vi "eyecat MAX v02_test.vi"() -> ()   [LabVIEW 2014]
doc: "This VI is an upgrade from the WIN 1_v4 that implements the ageing subrutine"
uses:
  Buttons/String output.ctl
  <vilib>/Utility/miscctls.llb/LVRowAndColumnTypeDef.ctl
  Buttons/Numeric control.ctl
  Buttons/String input.ctl
  Buttons/Numeric indicator.ctl
  Controls Win/Control 3.ctl
  <vilib>/Platform/TimedLoop/XDataNode/nitl_modes.ctl
  <vilib>/Platform/TimedLoop/XDataNode/timing_clust.ctl
  <vilib>/Platform/TimedLoop/XDataNode/wakeup.ctl
  <vilib>/Utility/file.llb/Read From Spreadsheet File (DBL).vi
  <vilib>/Utility/file.llb/Write To Spreadsheet File (string).vi
  <vilib>/Utility/file.llb/Read From Spreadsheet File (string).vi
  <vilib>/regexp/Match Regular Expression.xnode
  <vilib>/Platform/TimedLoop/XDataNode/XDataNode.xnode
  <vilib>/Platform/TimedLoop/XDataNode/XDNodeRunTimeDep.lvlib
panel:
  out "output cluster":T2
  out "Lambda":dbl[](array[numeric])
  out "MKS HC":dbl
  in  "HC Index":i32
  in  "MFC Number":i32
  out "Open/Closed Loop array":dbl[](array[numeric])
  out "Air Cyc 2 array":dbl[](array[numeric])
  in  "Cycle size":i32
  out "MFC Setpoint/Delivery":dynamicdata(graph)
  out "ExtAnDn":bool
  out "ExtAnUp":bool
  out "HC Cyc 2 Array":dbl[](array[numeric])
  out "SO Valve 2 array":dbl[](array[numeric])
  out "SO Valve 1 array":dbl[](array[numeric])
  out "Air Bal array":dbl[](array[numeric])
  out "HC Bal array":dbl[](array[numeric])
  out "Air Cyc 1 array":dbl[](array[numeric])
  out "HC Cyc 1 array":dbl[](array[numeric])
  out "File name":string
  out "Log?":bool
  out "Advanced Logging":bool
  out "Connected":bool
  out "MKS 1":i16
  out "MKS 2":i16
  out "Furnace temp 2":dbl
  out "Full system?":bool
  out "Log interval (seconds)":T1
  in  "Flow rate Age":dbl
  in  "Inlet temp Age":dbl
  out "Stopped?":bool
  in  "Stop Cmd":T1
  out "Connected?":bool
  out "Error":dbl
  out "Iteration Duration":i64
  out "Finished Late? [i-1]":bool
  in  "stop TCP":bool
  in  "SO2 ppm":dbl
  out "Furnace temp 1":dbl
  out "stop 2":bool
  in  "Enum 1":i16=1
  in  "Acknowledge":bool
  out "Test number":u16
  out "Flag1":bool=TRUE
  out "EditPos Subc":T3
  out "Flag 2":bool=TRUE
  in  "Tab Control":T4(tab)
  out "Doors Unlocked":bool
  in  "Temperature Limit (°C)":T1=800.0 min=0.0 max=1200.0 step=1.0
  in  "Log Test Button":bool
  in  "File Name":T5="Test"
  in  "File Path":path=path "C:/DATA LOG"
  out "Fail":bool
  out "Pass":bool
  in  "Select Test Type":T6(radio)
  out "Standby":bool
  out "Doors Open":bool
  out "Extractor Fan On":bool
  out "Test In Progress":bool
  out "Cool Down":bool
  out "System Alarm":bool
  in  "Execute Leak Test Button":bool
  in  "Stop Test Button":bool
  in  "Start Test Button":bool
  in  "Advanced settings":bool
  in  "Inlet Temperature (°C)":T1=400.0 min=350.0 max=1000.0 step=1.0
  in  "Inlet LAMBDA Rich":T1=0.9 min=0.85 max=0.96 step=0.001
  in  "Inlet LAMBDA Lean":T1=1.2 min=1.02 max=3.0 step=0.001
  in  "Test Stop temperature (°C)":T1=300.0 min=100.0 max=1000.0 step=1.0
  in  "Test Start Temperature (°C)":T1=125.0 min=0.0 max=500.0 step=1.0
  in  "Furnace Ramp Rate (°C/min)":T1=15.0 min=1.0 max=50.0 step=0.1
  in  "NO:CO Ratio":T1=1.1 min=1.0 max=5.0 step=0.1
  in  "Inlet O2 (%)":T1=0.5 min=0.0 max=14.0 step=0.01
  in  "Inlet LAMBDA":T1=1.0 min=0.6 max=3.0 step=0.001
  out "Space Velocity (h-1)":T7
  out "Vol Flow @ STP (l/min)":T7
  in  "Test Flow Rate(g/s)":T1 min=0.0 max=100.0 step=0.01
  out "Sample Volume (litres)":T7
  in  "Number of Samples":T1=1.0 min=1.0 max=6.0 step=1.0
  in  "Sample Diameter (mm)":T1
  out "CO Theory (%)":T7 format="%#_3g"
  out "CO Theory (%)":T7 format="%#_3g"
  out "HC Theory (%)":T7
  in  "Sample Length (mm)":T1 min=0.0 step=0.5
  in  "NO ppm SW":dbl=500.0 caption="NO (ppm)" min=0.0 max=500.0 step=1.0
  in  "NO ppm Loff":T1 caption="NO ppm"
  in  "Delete sCycle":bool
  in  "Load sCycle":bool
  in  "Save sCycle":bool
  in  "Clear subcycle":bool
  in  "Clear Cycle Pattern":bool
  in  "Save Cycle":bool
  in  "Load Cycle":bool
  in  "Delete Cycle":bool
  out "Test Compiled":bool
  in  "Compile Test Button":bool
  in  "Sub-Cycle List":i32(listbox)=1
  in  "Cycle List":i32(listbox)=2
  out "Total Test Duration (hrs)":T8
  in  "Ageing Gas":enum32{"Radio Selection 1", "Radio Selection 2"}(radio)
  in  "Sub-Cycle Pattern":string[][](table) caption="Subcycle pattern"
  in  "Total Number of Cycles":T1=1.0 min=1.0 max=10000.0 step=1.0
  in  "Cycle Pattern":string[][](table)
  in  "Sub-Cycle Name":T5
  in  "Cycle Name":T5
  out "Heat Exchanger Temperatures (°C)":dynamicdata(graph)
  out "Flow Rate (g/s)":dynamicdata(graph)
  out "Sample Temperatures (°C)":dynamicdata(graph)
  out "System Temperatures (°C)":dynamicdata(graph)
  out "HC Concentration (ppm)":dynamicdata(graph)
  out "Lambda":dynamicdata(graph)
  out "M584L Upstream & Downstream":dynamicdata(graph)
  out "NO Concentration (ppm)":dynamicdata(graph)
  in  "Purge System":bool
  in  "Alarm ack":bool
  in  "Clear log":bool
  out "Table":string[][](table)
  out "Soft Alarm":bool
  out "Hard Alarm":bool
  # "0 HC Cyc 1\n1 Air Cyc 1\n2 Air Bal\n3 HC Bal\n4 Air Cyc 2\n5 HC Cyc 2"
  # "Test Type"
  # "Test Commands"
  # "System Indicators"
  # "Leak Test"
  # "Catalyst Specification"
  # "Lightoff Settings"
  # "Furnace Lightoff Settings"
  # "Sweep Settings"
  # "CO/HC Lightoff Settings"
  # "0.96 < lambda < 0.85"
  # "1.02< lambda < 1.6"
  # "350 < Tinlet < 1000"
  # "NO Lightoff Settings"
  # "Flow Specification"
  # "Cycle Compiled"
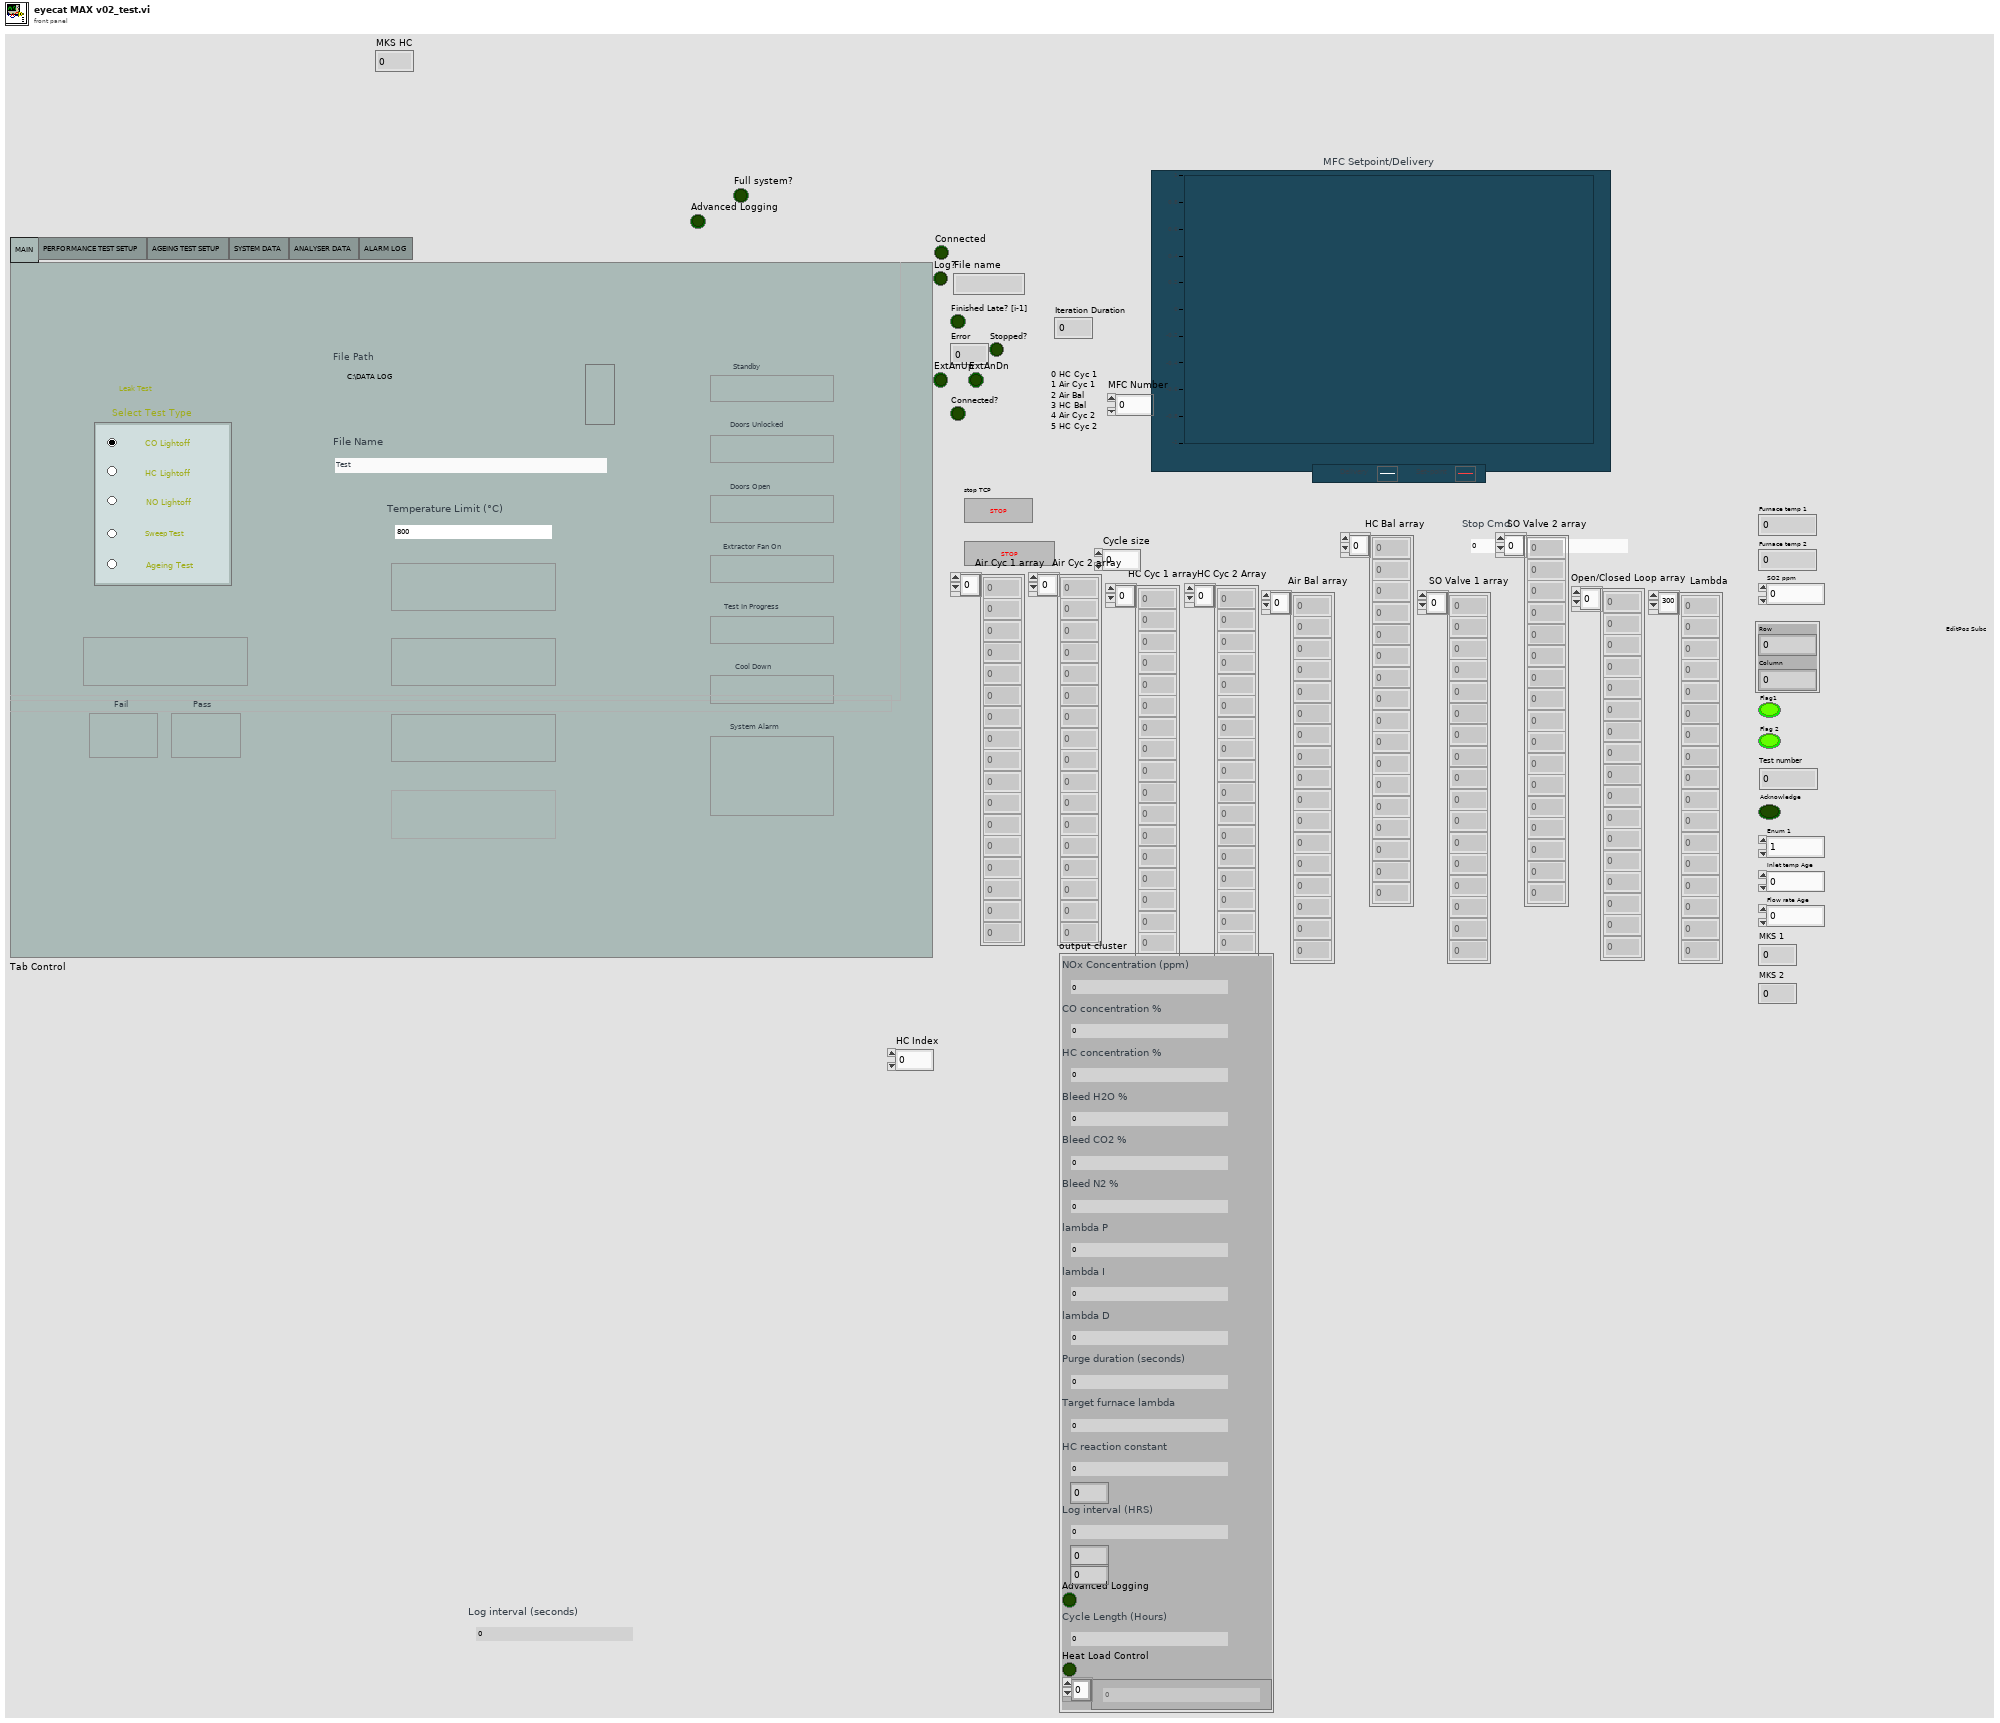
[diagram p1: front panel]
types:
  T1 = typedef "Numeric control.ctl" = dbl
  T2 = cluster{"NOx Concentration (ppm)":T1, "CO concentration %":T1, "HC concentration %":T1, "Bleed H2O %":T1, "Bleed CO2 %":T1, "Bleed N2 %":T1, "lambda P":T1, "lambda I":T1, "lambda D":T1, "Purge duration (seconds)":T1, "Target furnace lambda":T1, "HC reaction constant":T1, i16, "Log interval (HRS)":T1, i16, i16, "Advanced Logging":bool, "Cycle Length (Hours)":T1, "Heat Load Control":bool, T1[]}
  T3 = typedef "LVRowAndColumnTypeDef.ctl" = cluster{"Row":i32, "Column":i32}
  T4 = enum32{"MAIN", "PERFORMANCE TEST SETUP", "AGEING TEST SETUP", "SYSTEM DATA", "ANALYSER DATA", "ALARM LOG"}
  T5 = typedef "String input.ctl" = string
  T6 = enum32{"CO Lightoff", "HC Lightoff", "NO Lightoff", "Sweep Test", "Ageing Test"}
  T7 = typedef "Numeric indicator.ctl" = dbl
  T8 = typedef "String output.ctl" = string
  T9 = typedef "XDNodeRunTimeDep.lvlib/nitl_modes.ctl" = enum32{"No Change", "Process missed periods, maintain original phase", "Discard missed periods, maintain original phase", "Process missed periods, ignore original phase", "Discard missed periods, ignore original phase"}
  T10 = typedef "Control 3.ctl" = enum16{"main", "start test", "save subc", "load subc", "delete subc", "clear table 1", "update list 1", "save cycle", "load cycle", "delete cycle", "clear table 2", "update list 2", "calc HC CO", "Total time calc", "update Cycle pattern ", "load cycle name", "convert to num", "load test array", "check scycle name", "check cycle name", "Multigas connect", "Multigas disconnect"}
  T11 = enum8{"Enabled", "Disabled", "Disabled and Grayed Out"}
  T12 = typedef "XDNodeRunTimeDep.lvlib/timing_clust.ctl" = cluster{"Expected End [f-1]":u64, "Actual End [f-1]":u64, "Finished Late? [f-1]":bool, "Expected End [i-1]":u64, "Actual End [i-1]":u64, "Finished Late? [i-1]":bool, "Expected Start [i]":u64, "Actual Start [i]":u64, "Expected Start [f]":u64, "Actual Start [f]":u64, "Source Name":string, "Structure Name":string, "Period":i64, "Deadline":i64, "Offset":i64, "Start":i64, "Priority":i32, "Timeout":i32, "Mode":T9, "Wakeup Reason":T13, "Error":errorcluster, "Source Type":string, "Secondary Source Type":string, "Global End Time":u64, "Global Start Time":u64, "Frame Duration":u64, "Iteration Duration":u64, "Assigned CPU":i32, "I/O Scan Engine Mode":u32}
  T13 = typedef "XDNodeRunTimeDep.lvlib/wakeup.ctl" = enum32{"Normal", "Aborted", "Asynchronous wakeup", "Timing source error", "Timed loop error", "Timeout"}
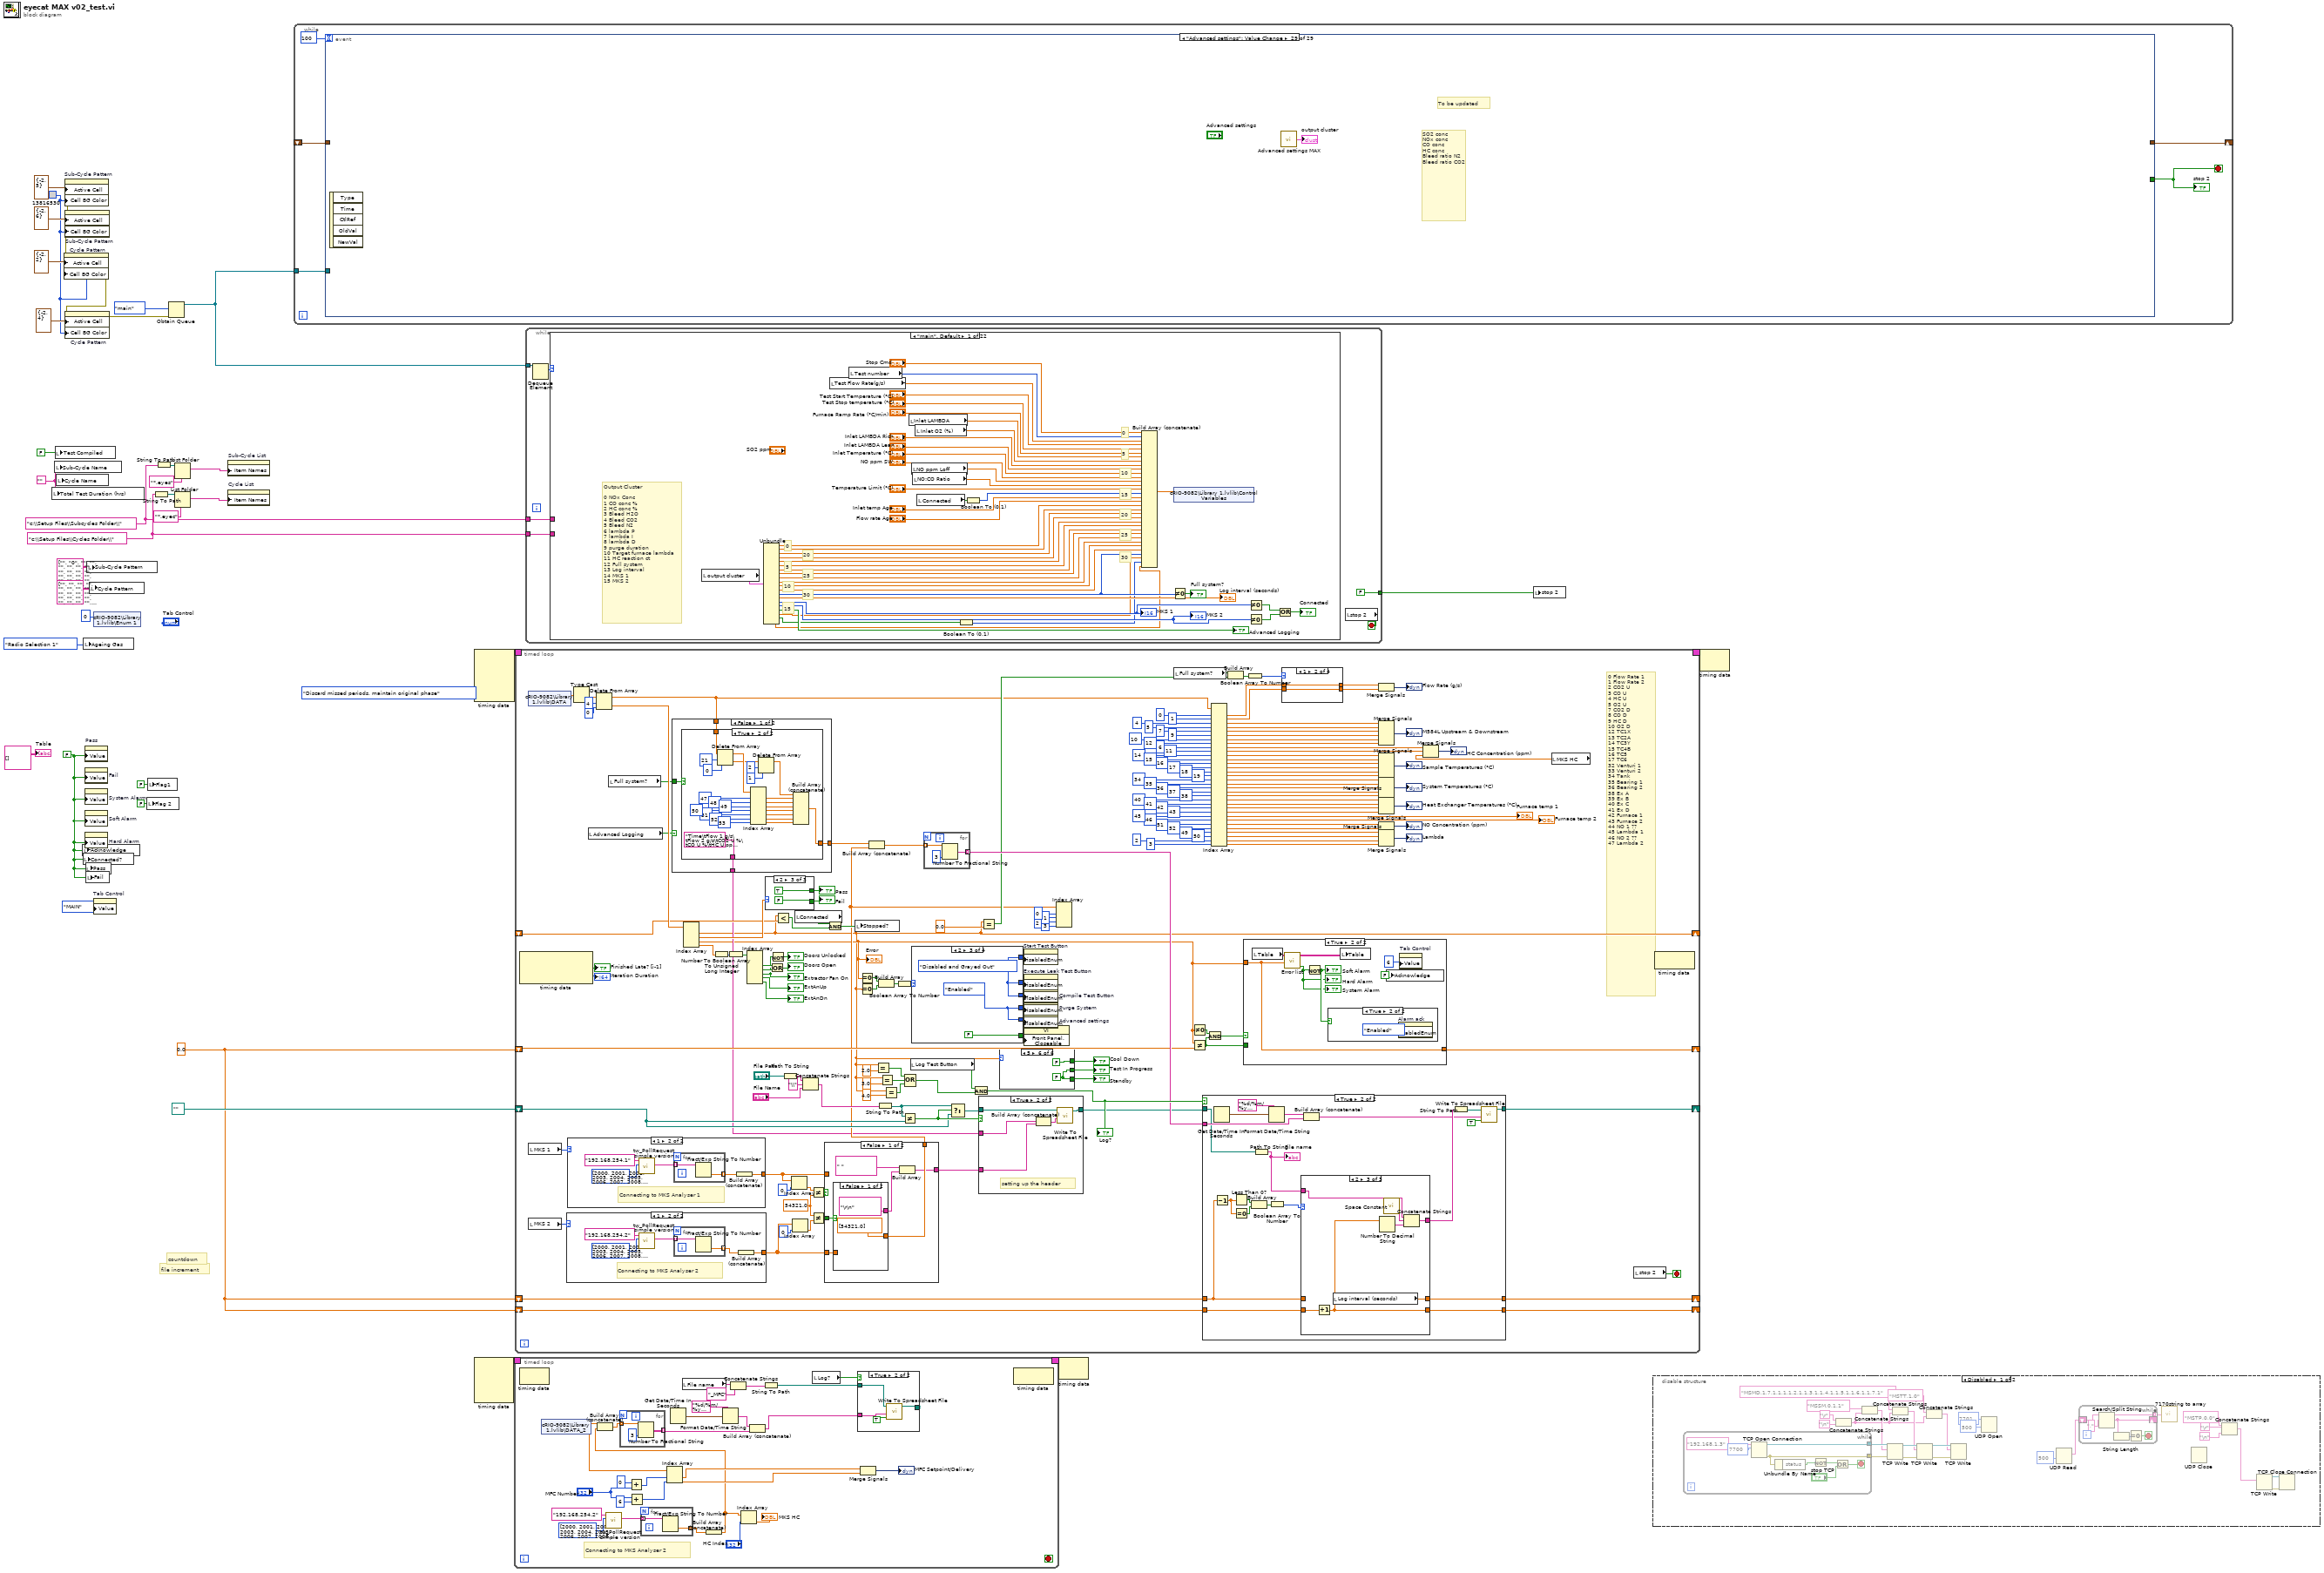
[diagram p0: block diagram]
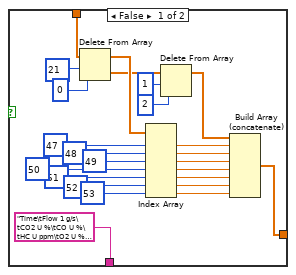
[diagram p4: hidden frame]
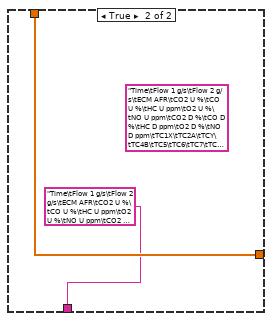
[diagram p5: hidden frame]
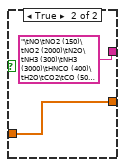
[diagram p6: hidden frame]
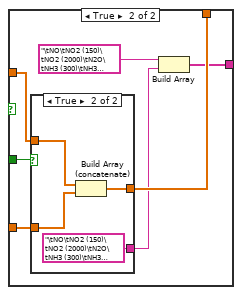
[diagram p7: hidden frame]
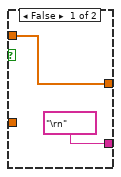
[diagram p8: hidden frame]
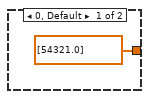
[diagram p9: hidden frame]
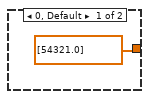
[diagram p10: hidden frame]
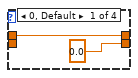
[diagram p11: hidden frame]
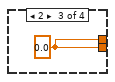
[diagram p12: hidden frame]
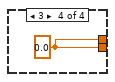
[diagram p13: hidden frame]
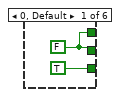
[diagram p14: hidden frame]
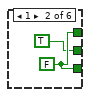
[diagram p15: hidden frame]
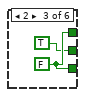
[diagram p16: hidden frame]
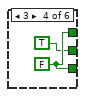
[diagram p17: hidden frame]
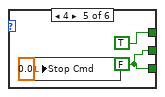
[diagram p18: hidden frame]
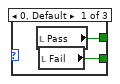
[diagram p19: hidden frame]
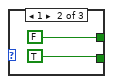
[diagram p20: hidden frame]
diagram:
  w4 = FALSE
  w3 = 0.0 ("y")
  w20 = ""
  w23 = "c:\\Setup Files\\Cycles Folder\\"
  w29 = u32 13816530
  w21 = "c:\\Setup Files\\Subcycles Folder\\"
  # "file increment"
  # "countdown"
  n1 = local write "Total Test Duration (hrs)"(w20) -> ()
  n2 = local write "Sub-Cycle Name"(w20) -> ()
  n3 = local write "Test Compiled"(FALSE ("Cycle Compiled")) -> ()
  n4 = local write "Cycle Name"(w20) -> ()
  n5 = property on="Sub-Cycle Pattern" class="Tbl (strict)"("Active Cell"=T3 {"Row"=-2, "Column"=5} ("Active Cell:Active Cell"), "Cell BG Color"=w29) -> (error out=w34:errorcluster)  [unwired: 2 in, 1 out]
  n6 = property on="Sub-Cycle Pattern" class="Tbl (strict)"(error in=w34, "Active Cell"=T3 {"Row"=-2, "Column"=6} ("Active Cell:Active Cell"), "Cell BG Color"=w29) -> (error out=w33:errorcluster)  [unwired: 1 in, 1 out]
  n7 = property on="Cycle Pattern" class="Tbl (strict)"(error in=w33, "Active Cell"=T3 {"Row"=-2, "Column"=2} ("Active Cell:Active Cell"), "Cell BG Color"=w29) -> (error out=w31:errorcluster)  [unwired: 1 in, 1 out]
  n8 = property on="Cycle Pattern" class="Tbl (strict)"(error in=w31, "Active Cell"=T3 {"Row"=-2, "Column"=4} ("Active Cell:Active Cell"), "Cell BG Color"=w29) -> (error out=w28:errorcluster)  [unwired: 1 in, 1 out]
  n9 = local write "Acknowledge"(w4) -> ()
  n10 = local write "Connected?"(w4) -> ()
  n11 = local write "Ageing Gas"(enum32{"Radio Selection 1", "Radio Selection 2"}."Radio Selection 1" ("Ageing Gas")) -> ()
  n12 = property on="Pass" class="Bool (strict)"("Value"=w4) -> ()  [unwired: 2 in, 2 out]
  n13 = property on="Fail" class="Bool (strict)"("Value"=w4) -> ()  [unwired: 2 in, 2 out]
  n14 = property on="System Alarm" class="Bool (strict)"("Value"=w4) -> ()  [unwired: 2 in, 2 out]
  n15 = property on="Soft Alarm" class="Bool (strict)"("Value"=w4) -> ()  [unwired: 2 in, 2 out]
  n16 = property on="Hard Alarm" class="Bool (strict)"("Value"=w4) -> ()  [unwired: 2 in, 2 out]
  n17 = local write "Pass"(w4) -> ()
  n18 = local write "Fail"(w4) -> ()
  n19 = local write "Sub-Cycle Pattern"(string[][] [["", "0", "", "", "", "", "", "", "", "", "", "", ""], ["", "", "", "", "", "", "", "", "", "", "", "", ""], ["", "", "", "", "", "", "", "", "", "", "", "", ""], ["", "", "", "", "", "", "", "", "", "", "", "", ""], ["", "", "", "", "", "", "", "", "", "", "", "", ""], ["", "", "", "", "", "", "", "", "", "", "", "", ""], ["", "", "", "", "", "", "", "", "", "", "", "", ""], ["", "", "", "", "", "", "", "", "", "", "", "", ""], ["", "", "", "", "", "", "", "", "", "", "", "", ""], ["", "", "", "", "", "", "", "", "", "", "", "", ""], ["", "", "", "", "", "", "", "", "", "", "", "", ""], ["", "", "", "", "", "", "", "", "", "", "", "", ""], ["", "", "", "", "", "", "", "", "", "", "", "", ""], ["", "", "", "", "", "", "", "", "", "", "", "", ""], ["", "", "", "", "", "", "", "", "", "", "", "", ""], ["", "", "", "", "", "", "", "", "", "", "", "", ""], ["", "", "", "", "", "", "", "", "", "", "", "", ""], ["", "", "", "", "", "", "", "", "", "", "", "", ""], ["", "", "", "", "", "", "", "", "", "", "", "", ""], ["", "", "", "", "", "", "", "", "", "", "", "", ""], ["", "", "", "", "", "", "", "", "", "", "", "", ""], ["", "", "", "", "", "", "", "", "", "", "", "", ""], ["", "", "", "", "", "", "", "", "", "", "", "", ""], ["", "", "", "", "", "", "", "", "", "", "", "", ""], ["", "", "", "", "", "", "", "", "", "", "", "", ""], ["", "", "", "", "", "", "", "", "", "", "", "", ""], ["", "", "", "", "", "", "", "", "", "", "", "", ""], ["", "", "", "", "", "", "", "", "", "", "", "", ""], ["", "", "", "", "", "", "", "", "", "", "", "", ""], ["", "", "", "", "", "", "", "", "", "", "", "", ""], ["", "", "", "", "", "", "", "", "", "", "", "", ""]]) -> ()
  n20 = local write "Cycle Pattern"(string[][] [["", "", "", "", ""], ["", "", "", "", ""], ["", "", "", "", ""], ["", "", "", "", ""], ["", "", "", "", ""], ["", "", "", "", ""], ["", "", "", "", ""], ["", "", "", "", ""], ["", "", "", "", ""], ["", "", "", "", ""], ["", "", "", "", ""], ["", "", "", "", ""], ["", "", "", "", ""], ["", "", "", "", ""], ["", "", "", "", ""], ["", "", "", "", ""], ["", "", "", "", ""], ["", "", "", "", ""], ["", "", "", "", ""], ["", "", "", "", ""], ["", "", "", "", ""], ["", "", "", "", ""], ["", "", "", "", ""], ["", "", "", "", ""], ["", "", "", "", ""], ["", "", "", "", ""], ["", "", "", "", ""], ["", "", "", "", ""], ["", "", "", "", ""], ["", "", "", "", ""], ["", "", "", "", ""]]) -> ()
  n21 = shared-variable "cRIO-9082\\Library 1.lvlib\\Enum 1"(u16 0 ("Enum 1")) -> ()  [unwired: 1 in, 1 out]
  n22 = property on="Tab Control" class="TabCtl (strict)"("Value"=T4."MAIN" ("Tab Control")) -> ()  [unwired: 2 in, 2 out]
  n23 = local write "Flag 2"(FALSE) -> ()
  n24 = local write "Flag1"(FALSE) -> ()
  n25 = String To Path(string=w23) -> (path=w24:path)
  n26 = String To Path(string=w21) -> (path=w26:path)
  n27 = Obtain Queue(element data type=Control_3."main" ("Enum"), error in (no error)=w28) -> (queue out=w37:refnum<queue>)  [unwired: 3 in, 2 out]
  n28 = List Folder(path=w24, pattern="*.eyec") -> (filenames=w25:string[])  [unwired: 2 in, 3 out]
  n29 = List Folder(path=w26, pattern="*.eyes") -> (filenames=w27:string[])  [unwired: 2 in, 3 out]
  n30 = property on="Sub-Cycle List" class="LstBox (strict)"("Item Names"=w27) -> ()  [unwired: 2 in, 2 out]
  n31 = property on="Cycle List" class="LstBox (strict)"("Item Names"=w25) -> ()  [unwired: 2 in, 2 out]
  n32 = while {
    tunnel: w37 -> [w43]
    shift-right: [w41] -> _
    shift-left: _ -> [w40]
    stop <- w39 stop-if-true
    n33 = event shown="[28] \"Advanced settings\": Value Change" {
      selector: _ -> [_ _ _ _ _ _ _ _ _ _ _ _ _ _ _ _ _ _ _ _ _ _ _ _ _ _ _ _ _]
      dyn-events: _ -> [_ _ _ _ _ _ _ _ _ _ _ _ _ _ _ _ _ _ _ _ _ _ _ _ _ _ _ _ _]
      timeout: 100 -> [_ _ _ _ _ _ _ _ _ _ _ _ _ _ _ _ _ _ _ _ _ _ _ _ _ _ _ _ _]
      tunnel: w43 -> [w46 w48 _ w57 w65 w72 w79 w90 w94 w105 w110 w113 w118 w140 w148 w149 _ _ _ _ w193 w209 _ w286 w304 _ w318 _ _]
      tunnel: [w44 w47 _ w58 w64 w71 w78 w89 w92 w100 w107 w112 w116 w137 _ _ _ _ _ _ _ _ _ _ _ _ _ _ _] -> w41
      tunnel: w40 -> [w44 w47 _ w58 w64 w71 w77 w89 w92 w100 w107 w112 w116 w137 _ _ _ _ _ _ _ _ _ _ _ _ _ _ _]
      tunnel: [_ _ w50 _ _ _ _ _ _ _ _ _ _ _ _ _ _ _ _ _ _ _ _ _ _ _ _ _ _] -> w39
      event Timeout {
        n34 = event-data() -> ()  [unwired: 1 in, 2 out]
        n35 = Enqueue Element(queue=w46, element=Control_3."main" ("Enum")) -> ()  [unwired: 2 in, 3 out]
      }
      event "Clear subcycle": Value Change {
        n36 = event-data() -> ()  [unwired: 1 in, 5 out]
        n37 = Enqueue Element(queue=w48, element=Control_3."clear table 1" ("Enum")) -> ()  [unwired: 2 in, 3 out]
      }
      event Panel Close? {
        n38 = event-data() -> ()  [unwired: 1 in, 3 out]
        n39 = Two Button Dialog(message="This command will close Eyecat!\nDo you wish to continue?", 1:"No" ("F button name (\"Cancel\")"), 2:"Yes" ("T button name (\"OK\")")) -> (T button?=w50:bool)
        n40 = Not(x=w50) -> (.not. x?=w51:bool)
        n41 = event-data("Discard?"=w51) -> ()  [unwired: 1 in, 1 out]
      }
      event "Save sCycle": Value Change {
        n42 = event-data() -> ()  [unwired: 1 in, 5 out]
        n43 = local read "Sub-Cycle Pattern"() -> (w55:string[][])
        n44 = call "Time column check.vi"("Array"=w55) -> ("Mistake?"=w56:bool)  [unwired: 10 in]
        n45 = case shown="False" w56 {
          tunnel: w57 -> [w59 _]
          frame False {
            n46 = Enqueue Element(queue=w59, element=Control_3."save subc") -> (queue out=w61:refnum<queue>)  [unwired: 2 in, 2 out]
            n47 = Enqueue Element(queue=w61, element=Control_3."update list 1") -> ()  [unwired: 2 in, 3 out]
          }
          frame True {
            n48 = One Button Dialog(message="The time sequence is incorrect!\nReview and save again!") -> ()  [unwired: 1 in, 1 out]
          }
        }
      }
      event "Load sCycle": Value Change {
        n49 = event-data() -> ()  [unwired: 1 in, 5 out]
        n50 = Enqueue Element(queue=w65, element=Control_3."load subc") -> ()  [unwired: 2 in, 3 out]
      }
      event "Delete sCycle": Value Change {
        n51 = event-data() -> ()  [unwired: 1 in, 5 out]
        n52 = Enqueue Element(queue=w72, element=Control_3."delete subc") -> (queue out=w74:refnum<queue>)  [unwired: 2 in, 2 out]
        n53 = Enqueue Element(queue=w74, element=Control_3."update list 1") -> (queue out=w70:refnum<queue>)  [unwired: 2 in, 2 out]
        n54 = Enqueue Element(queue=w70, element=Control_3."update Cycle pattern ") -> (queue out=w67:refnum<queue>)  [unwired: 2 in, 2 out]
        n55 = Enqueue Element(queue=w67, element=Control_3."Total time calc") -> ()  [unwired: 2 in, 3 out]
      }
      event "Sub-Cycle Pattern": Mouse Down; "Sub-Cycle Pattern": Value Change {
        n56 = event-data() -> ()  [unwired: 1 in, 3 out]
        n57 = property on="Sub-Cycle Pattern" class="Tbl (strict)"() -> ("EditPos"=w78:T3)  [unwired: 2 in, 2 out]
        n58 = Unbundle By Name(w78) -> ("Row"=w80:i32)  [unwired: 1 out]
        n59 = Less?(x=w80, y=30) -> (x < y?=w82:bool)
        n60 = case shown="True" w82 {
          tunnel: w79 -> [_ w87]
          frame False {
            n61 = One Button Dialog(message="This table is limited to 30 entries!") -> ()  [unwired: 1 in, 1 out]
          }
          frame True {
            n62 = Enqueue Element(queue=w87, element=Control_3."convert to num") -> (queue out=w86:refnum<queue>)  [unwired: 2 in, 2 out]
            n63 = Enqueue Element(queue=w86, element=Control_3."calc HC CO") -> ()  [unwired: 2 in, 3 out]
          }
        }
        "EditPos Subc" <- w77
        "Flag1" <- TRUE
      }
      event "Clear Cycle Pattern": Value Change {
        n64 = event-data() -> ()  [unwired: 1 in, 5 out]
        n65 = Enqueue Element(queue=w90, element=Control_3."clear table 2" ("Enum")) -> ()  [unwired: 2 in, 3 out]
        n66 = local write "Test Compiled"(FALSE ("Test Compiled")) -> ()
      }
      event "Save Cycle": Value Change {
        n67 = event-data() -> ()  [unwired: 1 in, 5 out]
        n68 = Enqueue Element(queue=w94, element=Control_3."update Cycle pattern ") -> (queue out=w93:refnum<queue>)  [unwired: 2 in, 2 out]
        n69 = Enqueue Element(queue=w93, element=Control_3."save cycle") -> (queue out=w97:refnum<queue>)  [unwired: 2 in, 2 out]
        n70 = Enqueue Element(queue=w97, element=Control_3."update list 2") -> ()  [unwired: 2 in, 3 out]
      }
      event "Load Cycle": Value Change {
        n71 = event-data() -> ()  [unwired: 1 in, 5 out]
        n72 = Enqueue Element(queue=w105, element=Control_3."load cycle") -> (queue out=w103:refnum<queue>)  [unwired: 2 in, 2 out]
        n73 = Enqueue Element(queue=w103, element=Control_3."update Cycle pattern ") -> (queue out=w102:refnum<queue>)  [unwired: 2 in, 2 out]
        n74 = local write "Test Compiled"(FALSE ("Test Compiled")) -> ()
        n75 = Enqueue Element(queue=w102, element=Control_3."Total time calc") -> ()  [unwired: 2 in, 3 out]
      }
      event "Delete Cycle": Value Change {
        n76 = event-data() -> ()  [unwired: 1 in, 5 out]
        n77 = Enqueue Element(queue=w110, element=Control_3."delete cycle") -> (queue out=w109:refnum<queue>)  [unwired: 2 in, 2 out]
        n78 = Enqueue Element(queue=w109, element=Control_3."update list 2") -> ()  [unwired: 2 in, 3 out]
      }
      event Value Change {
        n79 = event-data() -> ()  [unwired: 1 in, 5 out]
        n80 = Enqueue Element(queue=w113, element=Control_3."Total time calc") -> ()  [unwired: 2 in, 3 out]
      }
      event "Cycle Pattern": Mouse Up; "Cycle Pattern": Value Change {
        n81 = event-data() -> ()  [unwired: 1 in, 3 out]
        n82 = property on="Cycle Pattern" class="Tbl (strict)"() -> ("EditPos"=w120:T3)  [unwired: 2 in, 2 out]
        n83 = Unbundle By Name(w120) -> ("Row"=w117:i32, "Column"=w122:i32)
        n84 = Less?(x=w117, y=30) -> (x < y?=w121:bool)
        n85 = case shown="True" w121 {
          tunnel: w122 -> [_ w124]
          tunnel: w118 -> [_ w127]
          frame False {
            n86 = One Button Dialog(message="This table is limited to 30 entries!") -> ()  [unwired: 1 in, 1 out]
          }
          frame True {
            n87 = Equal?(x=w124, y=1) -> (x = y?=w128:bool)
            n88 = case shown="True" w128 {
              tunnel: w127 -> [w131 w134]
              tunnel: [w130 w133] -> w126
              frame False {
                n89 = Enqueue Element(queue=w131, element=Control_3."update Cycle pattern ") -> (queue out=w130:refnum<queue>)  [unwired: 2 in, 2 out]
              }
              frame True {
                n90 = Enqueue Element(queue=w134, element=Control_3."load cycle name") -> (queue out=w133:refnum<queue>)  [unwired: 2 in, 2 out]
              }
            }
            n91 = Enqueue Element(queue=w126, element=Control_3."Total time calc") -> ()  [unwired: 2 in, 3 out]
          }
        }
        "Flag 2" <- TRUE
      }
      event "Compile Test Button": Value Change {
        n92 = event-data() -> ()  [unwired: 1 in, 5 out]
        n93 = local read "Flag 2"() -> (w136:bool)
        n94 = case shown="True" w136 {
          tunnel: w140 -> [w141 w145]
          tunnel: [w141 w142] -> w138
          frame False {
          }
          frame True {
            n95 = Enqueue Element(queue=w145, element=Control_3."save cycle") -> (queue out=w143:refnum<queue>)  [unwired: 2 in, 2 out]
            n96 = Enqueue Element(queue=w143, element=Control_3."update list 2") -> (queue out=w142:refnum<queue>)  [unwired: 2 in, 2 out]
          }
        }
        n97 = Enqueue Element(queue=w138, element=Control_3."load test array") -> ()  [unwired: 2 in, 3 out]
      }
      event Value Change {
        n98 = event-data() -> ()  [unwired: 1 in, 5 out]
        n99 = Enqueue Element(queue=w148, element=Control_3."check scycle name") -> ()  [unwired: 2 in, 3 out]
      }
      event Value Change {
        n100 = event-data() -> ()  [unwired: 1 in, 5 out]
        n101 = Enqueue Element(queue=w149, element=Control_3."check cycle name") -> ()  [unwired: 2 in, 3 out]
      }
      event Value Change {
        n102 = event-data() -> ()  [unwired: 1 in, 5 out]
        n103 = Square(x="Sample Diameter (mm)") -> (x^2=w158:T1)
        n104 = Compound Arithmetic op=MULTIPLY(w158, "Sample Length (mm)", "Number of Samples", 3.141592653589793) -> (w157:T1)
        n105 = Divide(x=w157, y=4000000.0) -> (x/y=→"Sample Volume (litres)":T1)
      }
      event Value Change {
        # "O2Eq"
        n106 = event-data() -> ()  [unwired: 1 in, 5 out]
        n107 = local write "Inlet LAMBDA"("Inlet LAMBDA") -> ()
        n108 = local write "Inlet O2 (%)"("Inlet O2 (%)") -> ()
        n109 = Decrement(x="Inlet LAMBDA") -> (x-1=w173:T1)
        n110 = Multiply(x=4.76, y="Inlet LAMBDA") -> (x*y=w169:T1)
        n111 = Multiply(x=w173, y=100.0) -> (x*y=w171:T1)
        n112 = Add(x=0.33, y=w169) -> (x+y=w167:T1)
        n113 = Divide(x=w171, y=w167) -> (x/y=w166:T1)
        n114 = Subtract(x="Inlet O2 (%)", y=w166) -> (x-y=w164:T1)
        n115 = Multiply(x=w164, y=2.0) -> (x*y=→"CO Theory (%)":T1)
        n116 = Divide(x=w164, y=4.5) -> (x/y=→"HC Theory (%)":T1)
      }
      event Value Change {
        n117 = event-data() -> ()  [unwired: 1 in, 5 out]
        n118 = local write "NO ppm Loff"("NO ppm Loff") -> ()
        n119 = local write "NO:CO Ratio"("NO:CO Ratio") -> ()
        n120 = Divide(x="NO ppm Loff", y=T1 10000.0) -> (x/y=w176:T1)
        n121 = Multiply(x="NO:CO Ratio", y=w176) -> (x*y=→"CO Theory (%)":T1)
      }
      event Value Change {
        n122 = event-data() -> ()  [unwired: 1 in, 5 out]
        n123 = local read "Sample Volume (litres)"() -> (w181:T7)
        n124 = Equal?(x=w181, y=0.0) -> (x = y?=w180:bool)
        n125 = case shown="False" w180 {
          tunnel: w181 -> [w186 _]
          tunnel: "Test Flow Rate(g/s)" -> [w183 _]
          frame False {
            w188 = 60.0 ("y")
            n126 = Multiply(x=w183, y=w188) -> (x*y=w190:T1)
            n127 = Divide(x=w190, y=1.2) -> (x/y=w185:T1)
            "Vol Flow @ STP (l/min)" <- w185
            n128 = Multiply(x=w185, y=w188) -> (x*y=w187:T1)
            n129 = Divide(x=w187, y=w186) -> (x/y=→"Space Velocity (h-1)":T1)
          }
          frame True {
            n130 = One Button Dialog(message="Review sample specification first!") -> ()  [unwired: 1 in, 1 out]
          }
        }
      }
      event "Execute Leak Test Button": Value Change {
        n131 = event-data() -> ()  [unwired: 1 in, 5 out]
        n132 = flat-sequence {
          tunnel: w193 -> [w196]
          tunnel: [w196] -> w192
          tunnel: w192 -> [w199]
          frame #0 {
            n133 = local write "Test number"(u16 5) -> ()
            n134 = local write "Enum 1"(u16 3 ("Test number")) -> ()
          }
          frame #1 {
            n135 = Enqueue Element(queue=w199, element=Control_3."main" ("Enum")) -> (queue out=w197:refnum<queue>)  [unwired: 2 in, 2 out]
            n136 = Enqueue Element(queue=w197, element=Control_3."start test" ("Enum")) -> ()  [unwired: 2 in, 3 out]
          }
        }
      }
      event "Start Test Button": Value Change {
        n137 = event-data() -> ()  [unwired: 1 in, 5 out]
        n138 = property on="Log Test Button" class="Bool (strict)"() -> ("Value"=w208:bool)  [unwired: 2 in, 2 out]
        n139 = Boolean To (0,1)(Boolean=w208) -> (0, 1=w207:i16)
        n140 = Equal To 0?(x=w207) -> (x = 0?=w206:bool)
        n141 = case shown="True" w206 {
          tunnel: [TRUE ("T button?") w263] -> w201
          frame False {
          }
          frame True {
            # "Log Data Check"
            n142 = Two Button Dialog(message="You are not currently logging data!\nDo you wish to continue?", 1:"No" ("T button name (\"OK\")"), 2:"Yes" ("T button name (\"OK\")")) -> (T button?=w263:bool)
          }
        }
        n143 = Equal?(x=2.0, y=2.0) -> (x = y?=w202:bool)
        n144 = And(x=w202, y=w201) -> (x .and. y?=w203:bool)
        n145 = case shown="True" w203 {
          frame False {
          }
          frame True {
            n146 = flat-sequence {
              tunnel: "Cycle size" -> [w221]
              tunnel: [w221] -> w219
              tunnel: w219 -> [w224]
              tunnel: [w224] -> w218
              tunnel: w218 -> [w227]
              tunnel: [w227] -> w217
              tunnel: w217 -> [w230]
              tunnel: [w230] -> w216
              tunnel: [w233] -> w220
              tunnel: w216 -> [w233]
              tunnel: [w236] -> w215
              tunnel: w220 -> [w236]
              tunnel: w215 -> [w239]
              tunnel: [w239] -> w213
              tunnel: w213 -> [w242]
              tunnel: [w242] -> w212
              tunnel: w212 -> [w245]
              tunnel: [w245] -> w211
              tunnel: w211 -> [w248]
              tunnel: [w248] -> w210
              tunnel: w210 -> [w260]
              frame #0 {
                n147 = call-poly <vilib>:"Read From Spreadsheet File.vi"() -> ("all rows"=w223:dbl[][])  [unwired: 7 in, 4 out]
                n148 = Reshape Array(w223, w221) -> (→"Air Cyc 1 array":dbl[])
              }
              frame #1 {
                n149 = call-poly <vilib>:"Read From Spreadsheet File.vi"() -> ("all rows"=w225:dbl[][])  [unwired: 7 in, 4 out]
                n150 = Reshape Array(w225, w224) -> (→"Air Cyc 2 array":dbl[])
              }
              frame #2 {
                n151 = call-poly <vilib>:"Read From Spreadsheet File.vi"() -> ("all rows"=w229:dbl[][])  [unwired: 7 in, 4 out]
                n152 = Reshape Array(w229, w227) -> (→"HC Cyc 1 array":dbl[])
              }
              frame #3 {
                n153 = call-poly <vilib>:"Read From Spreadsheet File.vi"() -> ("all rows"=w232:dbl[][])  [unwired: 7 in, 4 out]
                n154 = Reshape Array(w232, w230) -> (→"HC Cyc 2 Array":dbl[])
              }
              frame #4 {
                n155 = call-poly <vilib>:"Read From Spreadsheet File.vi"() -> ("all rows"=w234:dbl[][])  [unwired: 7 in, 4 out]
                n156 = Reshape Array(w234, w233) -> (→"Air Bal array":dbl[])
              }
              frame #5 {
                n157 = call-poly <vilib>:"Read From Spreadsheet File.vi"() -> ("all rows"=w238:dbl[][])  [unwired: 7 in, 4 out]
                n158 = Reshape Array(w238, w236) -> (→"HC Bal array":dbl[])
              }
              frame #6 {
                n159 = call-poly <vilib>:"Read From Spreadsheet File.vi"() -> ("all rows"=w240:dbl[][])  [unwired: 7 in, 4 out]
                n160 = Reshape Array(w240, w239) -> (→"SO Valve 1 array":dbl[])
              }
              frame #7 {
                n161 = call-poly <vilib>:"Read From Spreadsheet File.vi"() -> ("all rows"=w243:dbl[][])  [unwired: 7 in, 4 out]
                n162 = Reshape Array(w243, w242) -> (→"SO Valve 2 array":dbl[])
              }
              frame #8 {
                n163 = call-poly <vilib>:"Read From Spreadsheet File.vi"() -> ("all rows"=w247:dbl[][])  [unwired: 7 in, 4 out]
                n164 = Reshape Array(w247, w245) -> (→"Open/Closed Loop array":dbl[])
              }
              frame #9 {
                n165 = local read "Open/Closed Loop array"() -> (w249:dbl[])
                n166 = local read "SO Valve 1 array"() -> (w251:dbl[])
                n167 = local read "SO Valve 2 array"() -> (w250:dbl[])
                n168 = local read "HC Cyc 2 Array"() -> (w255:dbl[])
                n169 = local read "HC Cyc 1 array"() -> (w254:dbl[])
                n170 = local read "Air Cyc 1 array"() -> (w252:dbl[])
                n171 = local read "Air Cyc 2 array"() -> (w253:dbl[])
                n172 = local read "HC Bal array"() -> (w257:dbl[])
                n173 = local read "Air Bal array"() -> (w256:dbl[])
                n174 = Build Array (concatenate)(w248, w252, w253, w254, w255, w256, w257, w251, w250, w249) -> (w258:dbl[])
                n175 = shared-variable "cRIO-9082\\Library 1.lvlib\\Inject_Arrays"(w258) -> ()  [unwired: 1 in, 1 out]
              }
              frame #10 {
                n176 = call-poly <vilib>:"Read From Spreadsheet File.vi"() -> ("all rows"=w261:dbl[][])  [unwired: 7 in, 4 out]
                n177 = Reshape Array(w261, w260) -> (w259:dbl[])
                "Lambda" <- w259
                n178 = shared-variable "cRIO-9082\\Library 1.lvlib\\Inject_Arrays_Lambda"(w259) -> ()  [unwired: 1 in, 1 out]
              }
            }
          }
        }
        n179 = case shown="True" w201 {
          tunnel: w209 -> [_ w268]
          frame False {
          }
          frame True {
            n180 = flat-sequence {
              tunnel: w268 -> [w271]
              tunnel: [w271] -> w267
              tunnel: w267 -> [w275]
              frame #0 {
                n181 = local write "Enum 1"(u16 1 ("Test number")) -> ()
                "Test number" <- "Select Test Type"
              }
              frame #1 {
                n182 = Enqueue Element(queue=w275, element=Control_3."main" ("Enum")) -> (queue out=w273:refnum<queue>)  [unwired: 2 in, 2 out]
                n183 = property on="Stop Test Button" class="Bool"("DisabledEnum"=T11."Enabled" ("Disabled")) -> ()  [unwired: 2 in, 2 out]
                n184 = Enqueue Element(queue=w273, element=Control_3."start test" ("Enum")) -> ()  [unwired: 2 in, 3 out]
              }
            }
          }
        }
      }
      event "Log Test Button": Value Change {
        n185 = event-data() -> ()  [unwired: 1 in, 6 out]
        n186 = property on="File Name" class="Str (strict)"() -> ("Value"=w279:T5)  [unwired: 2 in, 2 out]
        n187 = String Length(string=w279) -> (length=w278:i32)
        n188 = Equal To 0?(x=w278) -> (x = 0?=w277:bool)
        n189 = case shown="True" w277 {
          frame False {
          }
          frame True {
            n190 = One Button Dialog(message="A filename has not been entered!") -> ()  [unwired: 1 in, 1 out]
          }
        }
      }
      event "Stop Test Button": Value Change {
        n191 = event-data() -> ()  [unwired: 1 in, 5 out]
        n192 = flat-sequence {
          tunnel: w286 -> [w288]
          tunnel: [w288] -> w285
          tunnel: [w287] -> w283
          tunnel: w285 -> [w292]
          tunnel: [w291] -> w284
          tunnel: w283 -> [w291]
          tunnel: [w290] -> w282
          tunnel: w284 -> [w296]
          tunnel: w282 -> [w295]
          tunnel: [T11."Disabled and Grayed Out" ("Disabled")] -> w281
          frame #0 {
            n193 = local read "Connected?"() -> (w287:bool)
            n194 = local write "Stop Cmd"(T1 1.0 ("Stop Cmd")) -> ()
          }
          frame #1 {
            n195 = Enqueue Element(queue=w292, element=Control_3."main" ("Enum")) -> (queue out=w290:refnum<queue>)  [unwired: 2 in, 2 out]
          }
          frame #2 {
            n196 = case shown="True" w296 {
              tunnel: w295 -> [w297 w300]
              tunnel: [w297 w299] -> _
              frame False {
              }
              frame True {
                n197 = local write "Connected?"(FALSE ("Connected?")) -> ()
                n198 = Enqueue Element(queue=w300, element=Control_3."Multigas disconnect" ("Enum")) -> (queue out=w299:refnum<queue>)  [unwired: 2 in, 2 out]
              }
            }
          }
        }
        n199 = property on="Stop Test Button" class="Bool"("DisabledEnum"=w281) -> ()  [unwired: 2 in, 2 out]
      }
      event "Stopped?": Value Change {
        n200 = event-data() -> ()  [unwired: 1 in, 5 out]
        n201 = flat-sequence {
          tunnel: w304 -> [w308]
          tunnel: [w307] -> w303
          tunnel: [w306] -> w302
          tunnel: w303 -> [w310]
          tunnel: w302 -> [w309]
          frame #0 {
            n202 = local read "Connected?"() -> (w306:bool)
            n203 = Enqueue Element(queue=w308, element=Control_3."main" ("Enum")) -> (queue out=w307:refnum<queue>)  [unwired: 2 in, 2 out]
          }
          frame #1 {
            n204 = case shown="True" w309 {
              tunnel: w310 -> [_ w311]
              frame False {
              }
              frame True {
                n205 = local write "Connected?"(FALSE ("Connected?")) -> ()
                n206 = Enqueue Element(queue=w311, element=Control_3."Multigas disconnect" ("Enum")) -> ()  [unwired: 2 in, 3 out]
              }
            }
          }
        }
      }
      event "Alarm ack": Value Change {
        # "system alarm - set to off"
        n207 = event-data() -> ()  [unwired: 1 in, 5 out]
        n208 = local write "Acknowledge"(TRUE ("Acknowledge")) -> ()
        n209 = property on="Soft Alarm" class="Bool (strict)"("Value"=FALSE ("Acknowledge")) -> ()  [unwired: 2 in, 2 out]
        n210 = property on="Alarm ack" class="Bool"("DisabledEnum"=T11."Disabled and Grayed Out" ("Disabled")) -> ()  [unwired: 2 in, 2 out]
      }
      event "Purge System": Value Change {
        n211 = event-data() -> ()  [unwired: 1 in, 5 out]
        n212 = flat-sequence {
          tunnel: w318 -> [w320]
          tunnel: [w320] -> w317
          tunnel: w317 -> [w321]
          frame #0 {
            n213 = local write "Enum 1"(u16 4 ("Test number")) -> ()
          }
          frame #1 {
            n214 = Enqueue Element(queue=w321, element=Control_3."start test" ("Enum")) -> ()  [unwired: 2 in, 3 out]
          }
        }
      }
      event "Clear log": Value Change {
        n215 = event-data() -> ()  [unwired: 1 in, 5 out]
        n216 = local write "Table"(string[][] [] ("Table")) -> ()
      }
      event "Advanced settings": Value Change {
        # "To be updated"
        # "SO2 conc\nNOx conc\nCO conc\nHC conc\nBleed ratio N2\nBleed ratio CO2"
        n217 = event-data() -> ()  [unwired: 1 in, 5 out]
        n218 = call "Advanced settings MAX.vi"() -> ("output cluster"=→"output cluster":T2)  [unwired: 1 in]
      }
    }
    "stop 2" <- w39
  }
  n219 = node-c288() -> (w2:T12)  [unwired: 4 in]
  n220 = node-c288(nitl_modes."Discard missed periods, maintain original phase" ("Mode")) -> (w9:T12)  [unwired: 4 in]
  n221 = timed-loop {
    timing: w2 -> [_]
    timing-out: [_] -> w1
    stop <- _ stop-if-true
    # "Connecting to MKS Analyser 2"
    n222 = node-c288() -> ()  [unwired: 1 in, 1 out]
    n223 = shared-variable "cRIO-9082\\Library 1.lvlib\\DATA_2"() -> (w329:dbl[])  [unwired: 1 in, 1 out]
    n224 = call "tw_PollRequest simple version.vi"("EVID list"=i32[] [2000, 2001, 2002, 2003, 2004, 2005, 2006, 2007, 2008, 2009, 2010, 2011, 2012, 2013, 2014, 2015, 2016, 2017], "IP_ADD [127.0.0.1]"="192.168.254.2") -> ("values out"=w332:string[])  [unwired: 7 in, 2 out]
    n225 = Add(x=0 ("index"), y="MFC Number") -> (x+y=w335:i32)
    n226 = Add(x="MFC Number", y=6) -> (x+y=w330:i32)
    n227 = for {
      tunnel: [w353] -> w334 mode=indexing
      tunnel: w332 -> [w352] mode=indexing
      n228 = Fract/Exp String To Number(string=w352) -> (number=w353:dbl)  [unwired: 3 in, 1 out]
    }
    n229 = Index Array(array=w329, index #1=w335, index #2=w330) -> (element #1=w341:dbl, element #2=w340:dbl)
    n230 = Get Date/Time In Seconds() -> (seconds since 1Jan1904=w347:timestamp)
    n231 = local read "File name"() -> (w351:string)
    n232 = Build Array (concatenate)(w334) -> (w327:dbl[])
    n233 = Build Array (concatenate)(w329, w327) -> (w328:dbl[])
    n234 = for {
      tunnel: w328 -> [w360] mode=indexing
      tunnel: [w359] -> w344 mode=indexing
      n235 = Number To Fractional String(number=w360, precision (6)=i16 3) -> (F-format string=w359:string)  [unwired: 2 in]
    }
    n236 = Format Date/Time String(time format string (%c)="%d/%m/%y %H:%M:%S", seconds (now)=w347) -> (date/time string=w345:string)  [unwired: 1 in]
    n237 = Concatenate Strings(w351, "_MFC" ("string")) -> (w349:string)
    n238 = Index Array(array=w327, index="HC Index") -> (element=→"MKS HC":dbl)
    n239 = Build Array (concatenate)(w345, w344) -> (w343:string[])
    n240 = String To Path(string=w349) -> (path=w346:path)
    n241 = local read "Log?"() -> (w342:bool)
    n242 = case shown="True" w342 {
      tunnel: w346 -> [w354 w357]
      tunnel: [w354 w355] -> _
      tunnel: w343 -> [_ w356]
      frame False {
      }
      frame True {
        n243 = call-poly <vilib>:"Write To Spreadsheet File.vi"("append to file? (new file:F)"=TRUE, "1D data"=w356, "file path (dialog if empty)"=w357) -> ("new file path (Not A Path if cancelled)"=w355:path)  [unwired: 5 in]
      }
    }
    n244 = Merge Signals(w341, w340) -> (→"MFC Setpoint/Delivery":dynamicdata)
    n245 = node-c288() -> ()  [unwired: 1 in, 1 out]
  }
  n246 = timed-loop {
    timing: w9 -> [_]
    timing-out: [_] -> w8
    shift-right: [w383] -> _
    shift-left: path "" -> [w511]
    shift-right: [w469] -> _
    shift-left: w3 -> [w510]
    shift-right: [w384] -> _
    shift-left: _ -> [w480]
    shift-right: [w459] -> _
    shift-left: w3 -> [w462]
    shift-right: [w460] -> _
    shift-left: w3 -> [w461]
    stop <- w509 stop-if-true
    w393 = 54321.0 ("y")
    # "0 Flow Rate 1\n1 Flow Rate 2\n2 CO2 U\n3 CO U\n4 HC U\n5 O2 U\n7 CO2 D\n8 CO D\n9 HC D\n10 O2 D\n12 TC1X\n13 TC2A\n14 TC3Y\n15 TC4B\n16 TC5\n17 TC6\n32 Venturi 1\n33 Venturi 2\n34 Tank\n35 Bearing 1\n36 Bearing 2\n38 Ex A\n39 Ex B\n40 Ex C\n41 Ex D\n42 Furnace 1\n43 Furnace 2\n44 NO 1 ?? \n45 Lambda 1\n46 NO 2 ??\n47 Lambda 2"
    n247 = node-c288() -> (→"Finished Late? [i-1]":bool, →"Iteration Duration":i64)  [unwired: 1 in, 1 out]
    n248 = shared-variable "cRIO-9082\\Library 1.lvlib\\DATA"() -> (w508:dbl[])  [unwired: 1 in, 1 out]
    n249 = local read "MKS 1"() -> (w403:i16)
    n250 = local read "MKS 2"() -> (w402:i16)
    n251 = case shown="1" w402 {
      tunnel: [dbl[] [54321.0] w621] -> w399
      frame 0, Default {
      }
      frame 1 {
        # "Connecting to MKS Analyser 2"
        n252 = call "tw_PollRequest simple version.vi"("EVID list"=i32[] [2000, 2001, 2002, 2003, 2004, 2005, 2006, 2007, 2008, 2009, 2010, 2011, 2012, 2013, 2014], "IP_ADD [127.0.0.1]"="192.168.254.2") -> ("values out"=w619:string[])  [unwired: 7 in, 2 out]
        n253 = for {
          tunnel: [w623] -> w617 mode=indexing
          tunnel: w619 -> [w622] mode=indexing
          n254 = Fract/Exp String To Number(string=w622) -> (number=w623:dbl)  [unwired: 3 in, 1 out]
        }
        n255 = Build Array (concatenate)(w617) -> (w621:dbl[])
      }
    }
    n256 = case shown="1" w403 {
      tunnel: [dbl[] [54321.0] w625] -> w401
      frame 0, Default {
      }
      frame 1 {
        # "Connecting to MKS Analyser 1"
        n257 = call "tw_PollRequest simple version.vi"("EVID list"=i32[] [2000, 2001, 2002, 2003, 2004, 2005, 2006, 2007, 2008, 2009, 2010, 2011, 2012, 2013, 2014], "IP_ADD [127.0.0.1]"="192.168.254.1") -> ("values out"=w628:string[])  [unwired: 7 in, 2 out]
        n258 = for {
          tunnel: [w631] -> w626 mode=indexing
          tunnel: w628 -> [w630] mode=indexing
          n259 = Fract/Exp String To Number(string=w630) -> (number=w631:dbl)  [unwired: 3 in, 1 out]
        }
        n260 = Build Array (concatenate)(w626) -> (w625:dbl[])
      }
    }
    n261 = Type Cast(type=w508, x=w508) -> (*(type *) &x=w519:dbl[])
    n262 = local read "Advanced Logging"() -> (w389:bool)
    n263 = Delete From Array(array=w519, length=4, index=0) -> (deleted portion=w516:dbl[], array with subset deleted=w366:dbl[])
    n264 = local read "Full system?"() -> (w380:bool)
    n265 = case shown="False" w389 {
      tunnel: [w541 w592] -> w390
      tunnel: w366 -> [w542 w592]
      tunnel: [w540 "Time\tFlow 1 g/s\tFlow 2 g/s\tECM AFR\tCO2 U %\tCO U %\tHC U ppm\tO2 U %\tNO U ppm\tCO2 D %\tCO D %\tHC D ppm\tO2 D %\tNO D ppm\tTC1X\tTC2A\tTCY\tTC4B\tTC5\tTC6\tTC7\tTC8\tTC9\tTC10\tTC11\tTC12\tTC13\tTC14\tTC15\tTC16\tTC17\tTC18\tTC19\tTC20\tTC Vent 1\tTC Vent 2\tTC Tank\tTC Fan B1\tTC Fan B2\tTC Cab\tTC Ex A\tTC Ex B\tTC Ex C\tTC Ex D\tTC MFC Box\tTC Furn 1\tTC Furn 2\tTank Pressure\tRapidox\tLambda 1\tLambda 2\tNOX 1 ppm\tNOX 2 ppm\tUEGO 1\tUEGO 2" ("Heading string 2")] -> w388
      tunnel: w380 -> [w539 _]
      frame False {
        n266 = case shown="True" w539 {
          tunnel: w542 -> [w557 w572]
          tunnel: [w548 w574] -> w541
          tunnel: ["Time\tFlow 1 g/s\tCO2 U %\tCO U %\tHC U ppm\tO2 U %\tNO U ppm\tCO2 D %\tCO D %\tHC D ppm\tO2 D %\tNO D ppm\tTC1X\tTC2A\tTCY\tTC4B\tTC5\tTC6\tTC7\tTC8\tRapidox\tLambda 1\tLambda 2\tNOX 1 ppm\tNOX 2 ppm\tUEGO 1\tUEGO 2" ("Heading string 2") "Time\tFlow 1 g/s\tFlow 2 g/s\tCO2 U %\tCO U %\tHC U ppm\tO2 U %\tNO U ppm\tCO2 D %\tCO D %\tHC D ppm\tO2 D %\tNO D ppm\tTC1X\tTC2A\tTCY\tTC4B\tTC5\tTC6\tTC7\tTC8\tRapidox\tLambda 1\tLambda 2\tNOX 1 ppm\tNOX 2 ppm\tUEGO 1\tUEGO 2" ("Heading string 2")] -> w540
          frame False {
            n267 = Delete From Array(array=w557, length=21, index=0) -> (deleted portion=w544:dbl[], array with subset deleted=w556:dbl[])
            n268 = Index Array(array=w556, index #1=47 ("index"), index #2=48 ("index"), index #3=49 ("index"), index #4=50 ("index"), index #5=51 ("index"), index #6=52 ("index"), index #7=53 ("index")) -> (element #1=w555:dbl, element #2=w554:dbl, element #3=w553:dbl, element #4=w552:dbl, element #5=w551:dbl, element #6=w550:dbl, element #7=w549:dbl)
            n269 = Delete From Array(array=w544, length=1, index=2) -> (array with subset deleted=w543:dbl[])  [unwired: 1 out]
            n270 = Build Array (concatenate)(w543, w555, w554, w553, w552, w551, w550, w549) -> (w548:dbl[])
          }
          frame True {
            n271 = Delete From Array(array=w572, length=21, index=0) -> (deleted portion=w569:dbl[], array with subset deleted=w573:dbl[])
            n272 = Index Array(array=w573, index #1=47 ("index"), index #2=48 ("index"), index #3=49 ("index"), index #4=50 ("index"), index #5=51 ("index"), index #6=52 ("index"), index #7=53 ("index")) -> (element #1=w581:dbl, element #2=w580:dbl, element #3=w579:dbl, element #4=w578:dbl, element #5=w577:dbl, element #6=w576:dbl, element #7=w575:dbl)
            n273 = Delete From Array(array=w569, length=2, index=1) -> (array with subset deleted=w567:dbl[])  [unwired: 1 out]
            n274 = Build Array (concatenate)(w567, w581, w580, w579, w578, w577, w576, w575) -> (w574:dbl[])
          }
        }
      }
      frame True {
        (unwired) "Time\tFlow 1 g/s\tFlow 2 g/s\tECM AFR\tCO2 U %\tCO U %\tHC U ppm\tO2 U %\tNO U ppm\tCO2 D %\tCO D %\tHC D ppm\tO2 D %\tNO D ppm\tTC1X\tTC2A\tTCY\tTC4B\tTC5\tTC6\tTC7\tTC8\tTC9\tTC10\tTC11\tTC12\tTC13\tTC14\tTC15\tTC16\tTC17\tTC18\tTC19\tTC20\tTC Vent 1\tTC Vent 2\tTC Fan B1\tTC Fan B2\tTC Cab\tTC Ex A\tTC Ex B\tTC Ex C\tTC Ex D\tTC Furn 1\tTC Furn 2\tNOX 1 ppm\tNLambda 1\tNOX 2 ppm\tNLambda 2\tEGO 1\tEGO 2\tEGO 3\tEGO 4\tCO2 U %\tCO U %\tHC U ppm\tO2 U %\tNO U ppm\tCO2 D %\tCO D %\tHC D ppm\tO2 D %\tNO D ppm\r\n" ("Heading string 2")
      }
    }
    n275 = Index Array(array=w516) -> (element #1=w384:dbl, element #2=w486:dbl, element #3=w386:dbl, element #4=w479:dbl)  [unwired: 4 in]
    "Error" <- w386
    n276 = To Unsigned Long Integer(number=w479) -> (unsigned 32bit integer=w478:u32)
    n277 = Number To Boolean Array(number=w478) -> (Boolean array=w498:bool[])
    n278 = Index Array(array=w498) -> (element #2=w496:bool, element #3=w495:bool, element #4=w475:bool, element #5=→"ExtAnUp":bool, element #6=→"ExtAnDn":bool)  [unwired: 6 in, 1 out]
    "Extractor Fan On" <- w475
    n279 = case shown="2" w486 {
      tunnel: [w651 TRUE FALSE] -> w485
      tunnel: [w652 FALSE TRUE] -> w484
      frame 0, Default {
        n280 = local read "Pass"() -> (w652:bool)
        n281 = local read "Fail"() -> (w651:bool)
      }
      frame 1 {
      }
      frame 2 {
      }
    }
    "Pass" <- w484
    "Fail" <- w485
    n282 = Or(x=w496, y=w495) -> (x .or. y?=→"Doors Open":bool)
    n283 = Not(x=w475) -> (.not. x?=→"Doors Unlocked":bool)
    n284 = Less?(x=w384, y=w480) -> (x < y?=w477:bool)
    n285 = Path To String(path="File Path") -> (string=w473:string)
    n286 = Index Array(array=w401, index=0) -> (element=w397:dbl)
    n287 = Index Array(array=w399, index=0) -> (element=w395:dbl)
    n288 = local read "Connected"() -> (w476:bool)
    n289 = Concatenate Strings(w473, "\\" ("string"), "File Name") -> (w404:string)
    n290 = Not Equal?(x=w397, y=w393) -> (x != y?=w396:bool)
    n291 = Not Equal?(x=w393, y=w395) -> (x != y?=w394:bool)
    n292 = case shown="False" w396 {
      tunnel: [w598 w609] -> w392
      tunnel: w399 -> [w597 w608]
      tunnel: w401 -> [_ w607]
      tunnel: w394 -> [w596 w606]
      tunnel: [w595 w603] -> w391
      frame False {
        n293 = case shown="False" w596 {
          tunnel: [dbl[] [54321.0] w602] -> w598
          tunnel: w597 -> [_ w602]
          tunnel: ["\r\n" ("Heading string 2") "\tNO\tNO2 (150)\tNO2 (2000)\tN2O\tNH3 (300)\tNH3 (3000)\tHNCO (400)\tH2O\tCO2\tCO (500)\tCO (1)\tCH4 (250)\tCH4 (3000)\tNOxP\tPropane\r\n" ("Heading string 2")] -> w593
          frame False {
          }
          frame True {
          }
        }
        n294 = Build Array(" " ("Heading string 2"), w593) -> (w595:string[])
      }
      frame True {
        n295 = case shown="True" w606 {
          tunnel: [w611 w615] -> w609
          tunnel: w608 -> [_ w614]
          tunnel: w607 -> [w611 w613]
          tunnel: ["\rn" ("Heading string 2") "\tNO\tNO2 (150)\tNO2 (2000)\tN2O\tNH3 (300)\tNH3 (3000)\tHNCO (400)\tH2O\tCO2\tCO (500)\tCO (1)\tCH4 (250)\tCH4 (3000)\tNOxP\tPropane\r" ("Heading string 2")] -> w604
          frame False {
          }
          frame True {
            n296 = Build Array (concatenate)(w613, w614) -> (w615:dbl[])
          }
        }
        n297 = Build Array("\tNO\tNO2 (150)\tNO2 (2000)\tN2O\tNH3 (300)\tNH3 (3000)\tHNCO (400)\tH2O\tCO2\tCO (500)\tCO (1)\tCH4 (250)\tCH4 (3000)\tNOxP\tPropane" ("Heading string 2"), w604) -> (w603:string[])
      }
    }
    n298 = And(x=w476, y=w477) -> (x .and. y?=w468:bool)
    n299 = local write "Stopped?"(w468) -> ()
    n300 = Equal To 0?(x=w386) -> (x = 0?=w387:bool)
    n301 = Equal To 0?(x=w384) -> (x = 0?=w385:bool)
    n302 = Build Array (concatenate)(w390, w392) -> (w512:dbl[])
    n303 = Equal?(x=w384, y=2.0) -> (x = y?=w412:bool)
    n304 = String To Path(string=w404) -> (path=w470:path)
    n305 = Build Array(w387, w385) -> (w492:bool[])
    n306 = Equal?(x=w384, y=3.0) -> (x = y?=w409:bool)
    n307 = Equal?(x=w384, y=4.0) -> (x = y?=w407:bool)
    n308 = Boolean Array To Number(Boolean array=w492) -> (number=w491:u32)
    n309 = Not Equal?(x=w470, y=w511) -> (x != y?=w521:bool)
    n310 = Compound Arithmetic op=OR(w412, w409, w407) -> (w411:bool)
    n311 = local read "Log Test Button"() -> (w405:bool)
    n312 = case shown="2" w491 {
      tunnel: [w676 w677 w682 w684] -> w493
      tunnel: [w676 w677 w682 w684] -> w490
      tunnel: [w676 w677 w682 w684] -> w489
      tunnel: [w676 w677 w680 w684] -> w488
      tunnel: [T11."Enabled" ("Disabled") T11."Enabled" ("Disabled") w680 w684] -> w487
      tunnel: [FALSE FALSE FALSE TRUE] -> w467
      frame 0, Default {
        w676 = T11."Disabled and Grayed Out" ("Disabled")
      }
      frame 1 {
        w677 = T11."Disabled and Grayed Out" ("Disabled")
      }
      frame 2 {
        w680 = T11."Enabled" ("Disabled")
        w682 = T11."Disabled and Grayed Out" ("Disabled")
      }
      frame 3 {
        w684 = T11."Enabled" ("Disabled")
        (unwired) T11."Disabled and Grayed Out" ("Disabled")
      }
    }
    n313 = for {
      tunnel: w512 -> [w692] mode=indexing
      tunnel: [w691] -> w523 mode=indexing
      n314 = Number To Fractional String(number=w692, precision (6)=i16 3) -> (F-format string=w691:string)  [unwired: 2 in]
    }
    n315 = Select(t=w470, s=w521, f=w511) -> (s? t:f=w522:path)
    n316 = And(x=w405, y=w411) -> (x .and. y?=w538:bool)
    "Log?" <- w538
    n317 = case shown="True" w521 {
      tunnel: w522 -> [w685 w690]
      tunnel: [w685 w689] -> w520
      tunnel: w391 -> [_ w687]
      tunnel: w388 -> [_ w686]
      frame False {
      }
      frame True {
        # "setting up the header"
        n318 = Build Array (concatenate)(w686, w687) -> (w688:string[])
        n319 = call-poly <vilib>:"Write To Spreadsheet File.vi"("1D data"=w688, "file path (dialog if empty)"=w690) -> ("new file path (Not A Path if cancelled)"=w689:path)  [unwired: 6 in]
      }
    }
    n320 = Equal?(x=w384, y=0.0) -> (x = y?=w456:bool)
    n321 = case shown="5" w384 {
      tunnel: [w638 w641 w643 w645 TRUE FALSE] -> w483
      tunnel: [w638 TRUE TRUE TRUE w647 w649] -> w482
      tunnel: [TRUE w641 w643 w645 w647 w649] -> w481
      frame 0, Default {
        w638 = FALSE
      }
      frame 1 {
        w641 = FALSE
      }
      frame 2 {
        w643 = FALSE
      }
      frame 3 {
        w645 = FALSE
      }
      frame 4 {
        w647 = FALSE
        n322 = local write "Stop Cmd"(T1 0.0 ("Stop Cmd")) -> ()
      }
      frame 5 {
        w649 = FALSE
      }
    }
    "Cool Down" <- w483
    "Test In Progress" <- w482
    "Standby" <- w481
    n323 = property class="VI"("Front Panel.Closeable"=w467) -> ()  [unwired: 2 in, 2 out]
    n324 = property on="Start Test Button" class="Bool"("DisabledEnum"=w493) -> ()  [unwired: 2 in, 2 out]
    n325 = property on="Execute Leak Test Button" class="Bool"("DisabledEnum"=w490) -> ()  [unwired: 2 in, 2 out]
    n326 = property on="Compile Test Button" class="Bool"("DisabledEnum"=w489) -> ()  [unwired: 2 in, 2 out]
    n327 = property on="Purge System" class="Bool"("DisabledEnum"=w488) -> ()  [unwired: 2 in, 2 out]
    n328 = property on="Advanced settings" class="Bool"("DisabledEnum"=w487) -> ()  [unwired: 2 in, 2 out]
    n329 = Index Array(array=w392, index #1=0 ("index"), index #2=1 ("index"), index #3=2 ("index"), index #4=3 ("index")) -> ()  [unwired: 4 out]
    n330 = local read "Full system?"() -> (w457:bool)
    n331 = Not Equal To 0?(x=w386) -> (x != 0?=w514:bool)
    n332 = Not Equal?(x=w386, y=w510) -> (x != y?=w513:bool)
    n333 = case shown="True" w538 {
      tunnel: w520 -> [w696 w704]
      tunnel: [w696 w716] -> w383
      tunnel: w523 -> [_ w712]
      tunnel: w462 -> [_ w705]
      tunnel: w461 -> [w695 w700]
      tunnel: [w695 w702] -> w460
      tunnel: [w694 w701] -> w459
      frame False {
        n334 = local read "Log interval (seconds)"() -> (w694:T1)
      }
      frame True {
        n335 = Get Date/Time In Seconds() -> (seconds since 1Jan1904=w713:timestamp)
        n336 = Decrement(x=w705) -> (x-1=w706:T1)
        n337 = Less Than 0?(x=w706) -> (x < 0?=w707:bool)
        n338 = Equal To 0?(x=w706) -> (x = 0?=w708:bool)
        n339 = Build Array(w707, w708) -> (w709:bool[])
        n340 = Path To String(path=w704) -> (string=w699:string)
        "File name" <- w699
        n341 = Format Date/Time String(time format string (%c)="%d/%m/%y %H:%M:%S", seconds (now)=w713) -> (date/time string=w714:string)  [unwired: 1 in]
        n342 = Boolean Array To Number(Boolean array=w709) -> (number=w710:u32)
        n343 = case shown="2" w710 {
          tunnel: w705 -> [w723 w724 _]
          tunnel: [w722 w724 w727] -> w701
          tunnel: w699 -> [w721 w726 w730]
          tunnel: [w718 w726 w728] -> w703
          tunnel: [w717 w725 w729] -> w702
          tunnel: w700 -> [w717 w725 w733]
          frame 0, Default {
            n344 = Number To Decimal String(number=w717) -> (decimal integer string=w719:string)  [unwired: 1 in]
            n345 = call <vilib>:"Space Constant.vi"() -> ("String"=w720:string)
            n346 = Decrement(x=w723) -> (x-1=w722:T1)
            n347 = Concatenate Strings(w721, w720, w719) -> (w718:string)
          }
          frame 1 {
          }
          frame 2 {
            n348 = Increment(x=w733) -> (x+1=w729:dbl)
            n349 = local read "Log interval (seconds)"() -> (w727:T1)
            n350 = Number To Decimal String(number=w729) -> (decimal integer string=w731:string)  [unwired: 1 in]
            n351 = call <vilib>:"Space Constant.vi"() -> ("String"=w732:string)
            n352 = Concatenate Strings(w730, w732, w731) -> (w728:string)
          }
        }
        n353 = Build Array (concatenate)(w714, w712) -> (w698:string[])
        n354 = String To Path(string=w703) -> (path=w697:path)
        n355 = call-poly <vilib>:"Write To Spreadsheet File.vi"("append to file? (new file:F)"=TRUE, "1D data"=w698, "file path (dialog if empty)"=w697) -> ("new file path (Not A Path if cancelled)"=w716:path)  [unwired: 5 in]
      }
    }
    n356 = And(x=w514, y=w513) -> (x .and. y?=w515:bool)
    n357 = Index Array(array=w366, index #1=0 ("index"), index #2=1 ("index"), index #3=4 ("index"), index #4=5 ("index"), index #5=7 ("index"), index #6=9 ("index"), index #7=10 ("index"), index #8=12 ("index"), index #9=6 ("index"), index #10=11 ("index"), index #11=14 ("index"), index #12=15 ("index"), index #13=16 ("index"), index #14=17 ("index"), index #15=18 ("index"), index #16=19 ("index"), index #17=34 ("index"), index #18=35 ("index"), index #19=36 ("index"), index #20=37 ("index"), index #21=38 ("index"), index #22=40 ("index"), index #23=41 ("index"), index #24=42 ("index"), index #25=43 ("index"), index #26=45 ("index"), index #27=46 ("index"), index #28=51 ("index"), index #29=52 ("index"), index #30=49 ("index"), index #31=50 ("index"), index #32=2 ("index"), index #33=3 ("index")) -> (element #1=w365:dbl, element #2=w364:dbl, element #3=w452:dbl, element #4=w451:dbl, element #5=w379:dbl, element #6=w378:dbl, element #7=w377:dbl, element #8=w376:dbl, element #9=w375:dbl, element #10=w374:dbl, element #11=w446:dbl, element #12=w445:dbl, element #13=w444:dbl, element #14=w443:dbl, element #15=w442:dbl, element #16=w441:dbl, element #17=w435:dbl, element #18=w434:dbl, element #19=w433:dbl, element #20=w432:dbl, element #21=w431:dbl, element #22=w426:dbl, element #23=w425:dbl, element #24=w424:dbl, element #25=w423:dbl, element #26=→"Furnace temp 1":dbl, element #27=→"Furnace temp 2":dbl, element #28=w416:dbl, element #29=w382:dbl, element #30=w381:dbl, element #31=w413:dbl, element #32=w368:dbl, element #33=w367:dbl)
    n358 = Build Array(w457, w456) -> (w458:bool[])
    n359 = case shown="True" w515 {
      tunnel: w386 -> [w658 w669]
      tunnel: w513 -> [w661 _]
      tunnel: [w657 w669] -> w469
      frame False {
        n360 = Equal To 0?(x=w658) -> (x = 0?=w662:bool)
        n361 = And(x=w662, y=w661) -> (x .and. y?=w660:bool)
        n362 = case shown="True" w660 {
          frame False {
          }
          frame True {
            w665 = FALSE ("Ack hard alarm!")
            n363 = property on="Hard Alarm" class="Bool (strict)"("Value"=w665) -> ()  [unwired: 2 in, 2 out]
            n364 = property on="System Alarm" class="Bool (strict)"("Value"=w665) -> ()  [unwired: 2 in, 2 out]
          }
        }
        n365 = case shown="False" "Acknowledge" {
          tunnel: [w663 0.0 ("Numeric")] -> w657
          tunnel: w658 -> [w663 _]
          frame False {
          }
          frame True {
          }
        }
      }
      frame True {
        n366 = local read "Table"() -> (w672:string[][])
        n367 = call "Error list.vi"("Error code"=w669, "Error array in"=w672) -> ("Hard alarm?"=w666:bool, "Error array out"=w671:string[][])  [unwired: 8 in]
        "Hard Alarm" <- w666
        "System Alarm" <- w666
        n368 = Not(x=w666) -> (.not. x?=w667:bool)
        "Soft Alarm" <- w667
        n369 = case shown="True" w667 {
          frame False {
          }
          frame True {
            n370 = property on="Alarm ack" class="Bool"("DisabledEnum"=T11."Enabled" ("Disabled")) -> ()  [unwired: 2 in, 2 out]
          }
        }
        n371 = local write "Table"(w671) -> ()
        n372 = local write "Acknowledge"(FALSE ("Acknowledge")) -> ()
        n373 = property on="Tab Control" class="TabCtl (strict)"("Value"=6) -> ()  [unwired: 2 in, 2 out]
      }
    }
    n374 = Boolean Array To Number(Boolean array=w458) -> (number=w455:u32)
    n375 = case shown="1" w455 {
      tunnel: w365 -> [w633 w635 _ _]
      tunnel: w364 -> [_ w634 _ _]
      tunnel: [w633 w635 w636 w637] -> w454
      tunnel: [0.0 ("y") w634 w636 w637] -> w453
      frame 0, Default {
      }
      frame 1 {
      }
      frame 2 {
        w636 = 0.0 ("y")
      }
      frame 3 {
        w637 = 0.0 ("y")
      }
    }
    n376 = Merge Signals(w454, w453) -> (→"Flow Rate (g/s)":dynamicdata)
    n377 = Merge Signals(w452, w451, w379, w378, w377, w376) -> (→"M584L Upstream & Downstream":dynamicdata)
    n378 = Merge Signals(w446, w445, w444, w443, w442, w441) -> (→"Sample Temperatures (°C)":dynamicdata)
    n379 = Merge Signals(w435, w434, w433, w432, w431) -> (→"System Temperatures (°C)":dynamicdata)
    n380 = Merge Signals(w426, w425, w424, w423) -> (→"Heat Exchanger Temperatures (°C)":dynamicdata)
    n381 = Merge Signals(w416, w382) -> (→"NO Concentration (ppm)":dynamicdata)
    n382 = Merge Signals(w381, w413, w368, w367) -> (→"Lambda":dynamicdata)
    n383 = local read "MKS HC"() -> (w371:dbl)
    n384 = Merge Signals(w375, w374, w371) -> (→"HC Concentration (ppm)":dynamicdata)
    n385 = local read "stop 2"() -> (w509:bool)
    n386 = node-c288() -> ()  [unwired: 1 in, 1 out]
  }
  n387 = while {
    tunnel: w37 -> [w742]
    tunnel: w21 -> [w740]
    tunnel: w23 -> [w739]
    tunnel: [FALSE ("stop 2")] -> w11
    stop <- w743 stop-if-true
    n388 = Dequeue Element(queue=w742) -> (element=w741:T10)  [unwired: 2 in, 3 out]
    n389 = case shown="\"main\", Default" w741 {
      tunnel: w740 -> [_ _ _ w798 w809 w845 w879 _ _ _ _ _ _ _ w1242 _ _ _ _ _ _ _]
      tunnel: w739 -> [_ _ _ _ _ _ _ _ w892 w907 w962 w1007 _ _ _ _ _ _ _ _ _ _]
      frame "main", Default {
        # "20"
        # "25"
        # "30"
        # "15"
        # "10"
        # "5"
        # "0"
        # "30"
        # "25"
        # "20"
        # "15"
        # "10"
        # "5"
        # "0"
        # "Output Cluster\n\n0 NOx Conc\n1 CO conc %\n2 HC conc %\n3 Bleed H2O \n4 Bleed CO2\n5 Bleed N2 \n6 lambda P\n7 lambda I\n8 lambda D\n9 purge duration\n10 Target furnace lambda\n11 HC reaction ct\n12 Full system\n13 Log interval\n14 MKS 1\n15 MKS 2"
        n390 = local read "output cluster"() -> (w772:T2)
        n391 = Unbundle(w772) -> ("NOx Concentration (ppm)"=w758:T1, "CO concentration %"=w757:T1, "HC concentration %"=w756:T1, "Bleed H2O %"=w755:T1, "Bleed CO2 %"=w754:T1, "Bleed N2 %"=w769:T1, "lambda P"=w768:T1, "lambda I"=w767:T1, "lambda D"=w770:T1, "Purge duration (seconds)"=w771:T1, "Target furnace lambda"=w763:T1, "HC reaction constant"=w762:T1, w764:i16, "Log interval (HRS)"=→"Log interval (seconds)":T1, w751:i16, w749:i16, "Advanced Logging"=→"Advanced Logging":bool, "Cycle Length (Hours)"=w747:T1, "Heat Load Control"=w745:bool, w746:T1[])
        "MKS 1" <- w751
        "MKS 2" <- w749
        n392 = local read "Test Flow Rate(g/s)"() -> (w784:T1)
        n393 = local read "Test number"() -> (w789:u16)
        n394 = local read "Inlet LAMBDA"() -> (w776:T1)
        n395 = local read "NO ppm Loff"() -> (w774:T1)
        n396 = local read "NO:CO Ratio"() -> (w773:T1)
        n397 = local read "Inlet O2 (%)"() -> (w775:T1)
        n398 = local read "Connected"() -> (w778:bool)
        n399 = Boolean To (0,1)(Boolean=w745) -> (0, 1=w744:i16)
        n400 = Boolean To (0,1)(Boolean=w778) -> (0, 1=w761:i16)
        n401 = Build Array (concatenate)("Stop Cmd", w789, w784, "Test Start Temperature (°C)", "Test Stop temperature (°C)", "Furnace Ramp Rate (°C/min)", w776, w775, "Inlet LAMBDA Rich", "Inlet LAMBDA Lean", "Inlet Temperature (°C)", "NO ppm SW", w774, w773, "Temperature Limit (°C)", w761, "Inlet temp Age", "Flow rate Age", w758, w757, w756, w755, w754, w769, w768, w767, w770, w771, w763, w762, w764, w747, w744, w746) -> (w780:T1[])
        n402 = Not Equal To 0?(x=w764) -> (x != 0?=→"Full system?":bool)
        n403 = shared-variable "cRIO-9082\\Library 1.lvlib\\Control Variables"(w780) -> ()  [unwired: 1 in, 1 out]
        n404 = Not Equal To 0?(x=w751) -> (x != 0?=w752:bool)
        n405 = Not Equal To 0?(x=w749) -> (x != 0?=w750:bool)
        n406 = Or(x=w752, y=w750) -> (x .or. y?=→"Connected":bool)
      }
      frame "start test" {
        w790 = FALSE
        n407 = property on="Pass" class="Bool (strict)"("Value"=w790) -> ()  [unwired: 2 in, 2 out]
        n408 = property on="Fail" class="Bool (strict)"("Value"=w790) -> ()  [unwired: 2 in, 2 out]
        n409 = local write "Pass"(w790) -> ()
        n410 = local write "Fail"(w790) -> ()
        n411 = shared-variable "cRIO-9082\\Library 1.lvlib\\Enum 1"("Enum 1") -> ()  [unwired: 1 in, 1 out]
      }
      frame "clear table 1" {
        n412 = property on="Sub-Cycle Name" class="Str (strict)"("Value"="" ("Subcycle name")) -> ()  [unwired: 2 in, 2 out]
        n413 = local write "Sub-Cycle Pattern"(string[][] [["", "0", "", "", "", "", "", "", "", "", "", "", ""], ["", "", "", "", "", "", "", "", "", "", "", "", ""], ["", "", "", "", "", "", "", "", "", "", "", "", ""], ["", "", "", "", "", "", "", "", "", "", "", "", ""], ["", "", "", "", "", "", "", "", "", "", "", "", ""], ["", "", "", "", "", "", "", "", "", "", "", "", ""], ["", "", "", "", "", "", "", "", "", "", "", "", ""], ["", "", "", "", "", "", "", "", "", "", "", "", ""], ["", "", "", "", "", "", "", "", "", "", "", "", ""], ["", "", "", "", "", "", "", "", "", "", "", "", ""], ["", "", "", "", "", "", "", "", "", "", "", "", ""], ["", "", "", "", "", "", "", "", "", "", "", "", ""], ["", "", "", "", "", "", "", "", "", "", "", "", ""], ["", "", "", "", "", "", "", "", "", "", "", "", ""], ["", "", "", "", "", "", "", "", "", "", "", "", ""], ["", "", "", "", "", "", "", "", "", "", "", "", ""], ["", "", "", "", "", "", "", "", "", "", "", "", ""], ["", "", "", "", "", "", "", "", "", "", "", "", ""], ["", "", "", "", "", "", "", "", "", "", "", "", ""], ["", "", "", "", "", "", "", "", "", "", "", "", ""], ["", "", "", "", "", "", "", "", "", "", "", "", ""], ["", "", "", "", "", "", "", "", "", "", "", "", ""], ["", "", "", "", "", "", "", "", "", "", "", "", ""], ["", "", "", "", "", "", "", "", "", "", "", "", ""], ["", "", "", "", "", "", "", "", "", "", "", "", ""], ["", "", "", "", "", "", "", "", "", "", "", "", ""], ["", "", "", "", "", "", "", "", "", "", "", "", ""], ["", "", "", "", "", "", "", "", "", "", "", "", ""], ["", "", "", "", "", "", "", "", "", "", "", "", ""], ["", "", "", "", "", "", "", "", "", "", "", "", ""], ["", "", "", "", "", "", "", "", "", "", "", "", ""]]) -> ()
        n414 = local write "Flag1"(FALSE) -> ()
      }
      frame "update list 1" {
        n415 = String To Path(string=w798) -> (path=w797:path)
        n416 = List Folder(path=w797, pattern="*.eyes") -> (filenames=w796:string[])  [unwired: 2 in, 3 out]
        n417 = property on="Sub-Cycle List" class="LstBox (strict)"("Item Names"=w796) -> ()  [unwired: 2 in, 2 out]
      }
      frame "save subc" {
        w802 = ".eyes" ("string")
        n418 = local read "Sub-Cycle Name"() -> (w801:T5)
        n419 = String To Path(string=w809) -> (path=w814:path)
        n420 = Equal?(x=w801, y="") -> (x = y?=w806:bool)
        n421 = List Folder(path=w814, pattern="*.eyes" ("string")) -> (filenames=w813:string[])  [unwired: 2 in, 3 out]
        n422 = Concatenate Strings(w801, w802) -> (w800:string)
        n423 = Concatenate Strings(w809, w801, w802) -> (w815:string)
        n424 = Search 1D Array(1D array=w813, element=w800) -> (index of element=w812:i32)  [unwired: 1 in]
        n425 = case shown="True" w806 {
          tunnel: [TRUE FALSE] -> w805
          frame False {
          }
          frame True {
            n426 = One Button Dialog(message="Insert file name!") -> ()  [unwired: 1 in, 1 out]
          }
        }
        n427 = String To Path(string=w815) -> (path=w808:path)
        n428 = Equal?(x=w812, y=-1) -> (x = y?=w810:bool)
        n429 = case shown="False" w810 {
          selector: w810 -> [_ w821]
          tunnel: [w819 w821] -> w804
          frame False {
            n430 = Two Button Dialog(message="A file with this name already exists!\nDo you want to overwrite?") -> (T button?=w819:bool)  [unwired: 2 in]
          }
          frame True {
          }
        }
        n431 = And(x=w804, y=w805) -> (x .and. y?=w803:bool)
        n432 = case shown="True" w803 {
          tunnel: w808 -> [_ w826]
          frame False {
          }
          frame True {
            n433 = local read "Sub-Cycle Pattern"() -> (w825:string[][])
            n434 = call "Table check.vi"("Input table"=w825) -> ("Incomplete?"=w823:bool, "Length"=w824:i32)  [unwired: 9 in]
            n435 = case shown="False" w823 {
              tunnel: w825 -> [w834 _]
              tunnel: w826 -> [w833 _]
              tunnel: w824 -> [w832 _]
              tunnel: string[] [] -> [w831 _]
              frame False {
                n436 = for {
                  N: w832 -> [_]
                  tunnel: w834 -> [w841]
                  shift-right: [w838] -> w830
                  shift-left: w831 -> [w839]
                  i -> [w840]
                  n437 = Index Array(array=w841, index (row)=w840) -> (element=w837:string[])  [unwired: 1 in]
                  n438 = Delete From Array(array=w837, index=0) -> (array with subset deleted=w836:string[])  [unwired: 1 in, 1 out]
                  n439 = Build Array (concatenate)(w839, w836) -> (w838:string[])
                }
                n440 = Build Array (concatenate)("SubCycle Data File for EYECAT - do not modify", w830) -> (w828:string[])
                n441 = call-poly <vilib>:"Write To Spreadsheet File.vi"("1D data"=w828, "file path (dialog if empty)"=w833) -> ()  [unwired: 6 in, 1 out]
              }
              frame True {
                n442 = One Button Dialog(message="The table is incomplete!\nplease review and save again!") -> ()  [unwired: 1 in, 1 out]
              }
            }
            n443 = local write "Flag1"(FALSE) -> ()
          }
        }
      }
      frame "load subc" {
        n444 = local read "Flag1"() -> (w846:bool)
        n445 = case shown="True" w846 {
          tunnel: [w873 w875] -> w844
          tunnel: w845 -> [w873 w875]
          tunnel: [TRUE w874] -> w843
          frame False {
          }
          frame True {
            n446 = Two Button Dialog(message="The table has been modified.\nDo you want to continue?") -> (T button?=w874:bool)  [unwired: 2 in]
          }
        }
        n447 = case shown="True" w843 {
          tunnel: w844 -> [_ w850]
          frame False {
          }
          frame True {
            n448 = property on="Sub-Cycle List" class="LstBox (strict)"() -> ("Item Names"=w862:string[])  [unwired: 2 in, 2 out]
            n449 = Index Array(array=w862, index="Sub-Cycle List") -> (element=w849:string)
            n450 = Concatenate Strings(w850, w849) -> (w860:string)
            n451 = Search/Split String(string=w849, search string/char (-)=".") -> (substring before match=w847:string)  [unwired: 1 in, 2 out]
            n452 = local write "Sub-Cycle Name"(w847) -> ()
            n453 = String To Path(string=w860) -> (path=w859:path)
            n454 = call-poly <vilib>:"Read From Spreadsheet File.vi"("file path (dialog if empty)"=w859) -> ("first row"=w855:string[])  [unwired: 6 in, 4 out]
            n455 = Delete From Array(array=w855, length=1, index=0) -> (array with subset deleted=w852:string[])  [unwired: 1 out]
            n456 = Array Size(array=w852) -> (size(s)=w858:i32)
            n457 = Divide(x=w858, y=12) -> (x/y=w851:dbl)
            n458 = for {
              N: w851 -> [_]
              shift-right: [w868] -> _
              shift-left: w852 -> [w871]
              tunnel: [w867] -> w856 mode=indexing
              i -> [w866]
              n459 = Increment(x=w866) -> (x+1=w865:i32)
              n460 = Delete From Array(array=w871, length=12, index=0) -> (deleted portion=w863:string[], array with subset deleted=w868:string[])
              n461 = Number To Decimal String(number=w865) -> (decimal integer string=w864:string)  [unwired: 1 in]
              n462 = Build Array (concatenate)(w864, w863) -> (w867:string[])
            }
            n463 = local write "Sub-Cycle Pattern"(w856) -> ()
          }
        }
      }
      frame "delete subc" {
        n464 = Two Button Dialog(message="This operation will permanently delete this file!\nDo you want to continue?") -> (T button?=w878:bool)  [unwired: 2 in]
        n465 = case shown="True" w878 {
          tunnel: w879 -> [_ w884]
          frame False {
          }
          frame True {
            n466 = local read "Sub-Cycle List"() -> (w881:i32)
            n467 = property on="Sub-Cycle List" class="LstBox (strict)"() -> ("Item Names"=w882:string[])  [unwired: 2 in, 2 out]
            n468 = Index Array(array=w882, index=w881) -> (element=w886:string)
            n469 = Concatenate Strings(w884, w886) -> (w885:string)
            n470 = local write "Flag1"(FALSE) -> ()
            n471 = String To Path(string=w885) -> (path=w883:path)
            n472 = Delete(path (use dialog)=w883) -> ()  [unwired: 4 in, 3 out]
          }
        }
      }
      frame "clear table 2" {
        n473 = property on="Cycle Name" class="Str (strict)"("Value"="" ("Subcycle name")) -> ()  [unwired: 2 in, 2 out]
        n474 = local write "Flag 2"(FALSE) -> ()
        n475 = local write "Cycle Pattern"(string[][] [["", "", "", "", ""], ["", "", "", "", ""], ["", "", "", "", ""], ["", "", "", "", ""], ["", "", "", "", ""], ["", "", "", "", ""], ["", "", "", "", ""], ["", "", "", "", ""], ["", "", "", "", ""], ["", "", "", "", ""], ["", "", "", "", ""], ["", "", "", "", ""], ["", "", "", "", ""], ["", "", "", "", ""], ["", "", "", "", ""], ["", "", "", "", ""], ["", "", "", "", ""], ["", "", "", "", ""], ["", "", "", "", ""], ["", "", "", "", ""], ["", "", "", "", ""], ["", "", "", "", ""], ["", "", "", "", ""], ["", "", "", "", ""], ["", "", "", "", ""], ["", "", "", "", ""], ["", "", "", "", ""], ["", "", "", "", ""], ["", "", "", "", ""], ["", "", "", "", ""], ["", "", "", "", ""]]) -> ()
      }
      frame "update list 2" {
        n476 = String To Path(string=w892) -> (path=w893:path)
        n477 = List Folder(path=w893, pattern="*.eyec") -> (filenames=w891:string[])  [unwired: 2 in, 3 out]
        n478 = property on="Cycle List" class="LstBox (strict)"("Item Names"=w891) -> ()  [unwired: 2 in, 2 out]
      }
      frame "save cycle" {
        w894 = ".eyec" ("string")
        n479 = local read "Cycle Name"() -> (w895:T5)
        n480 = String To Path(string=w907) -> (path=w908:path)
        n481 = List Folder(path=w908, pattern="*.eyec" ("string")) -> (filenames=w906:string[])  [unwired: 2 in, 3 out]
        n482 = Equal?(x=w895, y="") -> (x = y?=w901:bool)
        n483 = Concatenate Strings(w895, w894) -> (w897:string)
        n484 = Search 1D Array(1D array=w906, element=w897) -> (index of element=w905:i32)  [unwired: 1 in]
        n485 = Concatenate Strings(w907, w895, w894) -> (w910:string)
        n486 = case shown="True" w901 {
          tunnel: [TRUE FALSE] -> w899
          frame False {
          }
          frame True {
            n487 = One Button Dialog(message="Insert file name!") -> ()  [unwired: 1 in, 1 out]
          }
        }
        n488 = String To Path(string=w910) -> (path=w909:path)
        n489 = Equal?(x=w905, y=-1) -> (x = y?=w903:bool)
        n490 = case shown="False" w903 {
          selector: w903 -> [_ w959]
          tunnel: [w957 w959] -> w900
          frame False {
            n491 = Two Button Dialog(message="A file with this name already exists!\nDo you want to overwrite?") -> (T button?=w957:bool)  [unwired: 2 in]
          }
          frame True {
          }
        }
        n492 = And(x=w900, y=w899) -> (x .and. y?=w898:bool)
        n493 = case shown="True" w898 {
          tunnel: w909 -> [_ w917]
          frame False {
          }
          frame True {
            n494 = local read "Cycle Pattern"() -> (w916:string[][])
            n495 = call "Table check.vi"("Input table"=w916) -> ("Incomplete?"=w914:bool, "Length"=w915:i32)  [unwired: 9 in]
            n496 = case shown="False" w914 {
              tunnel: w917 -> [w926 _]
              tunnel: w916 -> [w925 _]
              tunnel: w915 -> [w918 _]
              frame False {
                n497 = Number To Decimal String(number=w918) -> (decimal integer string=w921:string)  [unwired: 1 in]
                n498 = for {
                  N: w918 -> [_]
                  tunnel: w925 -> [w955]
                  shift-right: [w943] -> w922
                  shift-left: string[] [] -> [w953]
                  i -> [w954]
                  w934 = 12 ("length")
                  n499 = Index Array(array=w955, index (row)=w954) -> (element=w949:string[])  [unwired: 1 in]
                  n500 = Index Array(array=w949, index=3) -> (element=w939:string)
                  n501 = Index Array(array=w949, index=1) -> (element=w938:string)
                  n502 = Concatenate Strings("C:\\Setup Files\\Subcycles Folder\\", w938) -> (w950:string)
                  n503 = String To Path(string=w950) -> (path=w951:path)
                  n504 = call-poly <vilib>:"Read From Spreadsheet File.vi"("file path (dialog if empty)"=w951) -> ("first row"=w942:string[])  [unwired: 6 in, 4 out]
                  n505 = Delete From Array(array=w942, length=1, index=0) -> (array with subset deleted=w936:string[])  [unwired: 1 out]
                  n506 = String Length(string=w936) -> (length=w945:i32[])
                  n507 = Array Size(array=w945) -> (size(s)=w937:i32)
                  n508 = Divide(x=w937, y=w934) -> (x/y=w935:dbl)
                  n509 = Decrement(x=w935) -> (x-1=w927:dbl)
                  n510 = Multiply(x=w934, y=w927) -> (x*y=w933:dbl)
                  n511 = Number To Decimal String(number=w927) -> (decimal integer string=w944:string)  [unwired: 1 in]
                  n512 = Delete From Array(array=w936, length=12, index=w933) -> (deleted portion=w930:string[], array with subset deleted=w931:string[])
                  n513 = Index Array(array=w930, index=0) -> (element=w928:string)
                  n514 = Build Array (concatenate)(w938, w939, w944, w928, w931) -> (w948:string[])
                  n515 = Build Array (concatenate)(w953, w948) -> (w943:string[])
                }
                n516 = local write "Flag 2"(FALSE) -> ()
                n517 = Build Array (concatenate)("Cycle Data File for EYECAT - do not modify", w921, w922) -> (w923:string[])
                n518 = call-poly <vilib>:"Write To Spreadsheet File.vi"("1D data"=w923, "file path (dialog if empty)"=w926) -> ()  [unwired: 6 in, 1 out]
              }
              frame True {
                n519 = One Button Dialog(message="The table is incomplete!\nplease review and save again!") -> ()  [unwired: 1 in, 1 out]
              }
            }
          }
        }
      }
      frame "load cycle" {
        n520 = local read "Flag 2"() -> (w963:bool)
        n521 = case shown="True" w963 {
          tunnel: [w1002 w1004] -> w960
          tunnel: w962 -> [w1002 w1004]
          tunnel: [TRUE ("T button?") w1003] -> w961
          frame False {
          }
          frame True {
            n522 = Two Button Dialog(message="The table has been modified.\nDo you want to continue?") -> (T button?=w1003:bool)  [unwired: 2 in]
          }
        }
        n523 = case shown="True" w961 {
          tunnel: w960 -> [_ w966]
          frame False {
          }
          frame True {
            n524 = property on="Cycle List" class="LstBox (strict)"() -> ("Item Names"=w982:string[])  [unwired: 2 in, 2 out]
            n525 = Index Array(array=w982, index="Cycle List") -> (element=w968:string)
            n526 = Concatenate Strings(w966, w968) -> (w981:string)
            n527 = Search/Split String(string=w968, search string/char (-)=".") -> (substring before match=w967:string)  [unwired: 1 in, 2 out]
            n528 = String To Path(string=w981) -> (path=w980:path)
            n529 = local write "Cycle Name"(w967) -> ()
            n530 = call-poly <vilib>:"Read From Spreadsheet File.vi"("file path (dialog if empty)"=w980) -> ("first row"=w964:string[])  [unwired: 6 in, 4 out]
            n531 = Delete From Array(array=w964, length=2, index=0) -> (array with subset deleted=w965:string[])  [unwired: 1 out]
            n532 = Index Array(array=w964, index=1) -> (element=w979:string)
            n533 = Decimal String To Number(string=w979) -> (number=w978:i32)  [unwired: 2 in, 1 out]
            n534 = for {
              N: w978 -> [_]
              tunnel: w965 -> [w1000]
              tunnel: [w995] -> w973 mode=indexing
              shift-right: [w985] -> _
              shift-left: 0 ("x") -> [w986]
              i -> [w999]
              w996 = ""
              n535 = Increment(x=w986) -> (x+1=w984:i32)
              n536 = Increment(x=w984) -> (x+1=w992:i32)
              n537 = Increment(x=w999) -> (x+1=w994:i32)
              n538 = Number To Decimal String(number=w994) -> (decimal integer string=w993:string)  [unwired: 1 in]
              n539 = Index Array(array=w1000, index #1=w986, index #2=w984, index #3=w992) -> (element #1=w998:string, element #2=w997:string, element #3=w991:string)
              n540 = Build Array(w993, w998, w996, w997, w996) -> (w995:string[])
              n541 = Decimal String To Number(string=w991) -> (number=w990:i32)  [unwired: 2 in, 1 out]
              n542 = Multiply(x=w990, y=12 ("x")) -> (x*y=w988:i32)
              n543 = Compound Arithmetic op=ADD(w988, 4, w986) -> (w985:i32)
            }
            n544 = Insert Into Array(array=string[][] [["", "", "", "", ""], ["", "", "", "", ""], ["", "", "", "", ""], ["", "", "", "", ""], ["", "", "", "", ""], ["", "", "", "", ""], ["", "", "", "", ""], ["", "", "", "", ""], ["", "", "", "", ""], ["", "", "", "", ""], ["", "", "", "", ""], ["", "", "", "", ""], ["", "", "", "", ""], ["", "", "", "", ""], ["", "", "", "", ""], ["", "", "", "", ""], ["", "", "", "", ""], ["", "", "", "", ""], ["", "", "", "", ""], ["", "", "", "", ""], ["", "", "", "", ""], ["", "", "", "", ""], ["", "", "", "", ""], ["", "", "", "", ""], ["", "", "", "", ""], ["", "", "", "", ""], ["", "", "", "", ""], ["", "", "", "", ""], ["", "", "", "", ""], ["", "", "", "", ""], ["", "", "", "", ""]], index (row)=0, new element=w973) -> (w972:string[][])  [unwired: 1 in]
            n545 = local write "Cycle Pattern"(w972) -> ()
          }
        }
      }
      frame "delete cycle" {
        n546 = Two Button Dialog(message="This operation will permanently delete this file!\nDo you want to continue?") -> (T button?=w1008:bool)  [unwired: 2 in]
        n547 = case shown="True" w1008 {
          tunnel: w1007 -> [_ w1013]
          frame False {
          }
          frame True {
            n548 = local read "Cycle List"() -> (w1014:i32)
            n549 = property on="Cycle List" class="LstBox (strict)"() -> ("Item Names"=w1015:string[])  [unwired: 2 in, 2 out]
            n550 = Index Array(array=w1015, index=w1014) -> (element=w1012:string)
            n551 = Concatenate Strings(w1013, w1012) -> (w1011:string)
            n552 = String To Path(string=w1011) -> (path=w1010:path)
            n553 = Delete(path (use dialog)=w1010) -> ()  [unwired: 4 in, 3 out]
            n554 = local write "Flag 2"(FALSE) -> ()
          }
        }
      }
      frame "calc HC CO" {
        n555 = local read "Sub-Cycle Pattern"() -> (w1032:string[][])
        n556 = Index Array(array=w1032, index (col) #1=3 ("disabled index (col)"), index (col) #2=4 ("index (col)"), index (col) #3=11 ("index (col)")) -> (element #1=w1022:string[], element #2=w1029:string[], element #3=w1016:string[])  [unwired: 3 in]
        n557 = Array Size(array=w1022) -> (size(s)=w1020:i32)
        n558 = Search 1D Array(1D array=w1022, element="") -> (index of element=w1019:i32)  [unwired: 1 in]
        n559 = Equal?(x=w1019, y=-1) -> (x = y?=w1021:bool)
        n560 = Select(t=w1020, s=w1021, f=w1019) -> (s? t:f=w1018:i32)
        n561 = for {
          N: w1018 -> [_]
          tunnel: [w1043] -> w1026 mode=indexing
          tunnel: [w1042] -> w1025 mode=indexing
          tunnel: w1022 -> [w1041] mode=indexing
          tunnel: w1029 -> [w1040] mode=indexing
          tunnel: w1016 -> [w1039] mode=indexing
          w1038 = ""
          n562 = Not Equal?(x=w1041, y=w1038) -> (x != y?=w1037:bool)
          n563 = Not Equal?(x=w1040, y=w1038) -> (x != y?=w1036:bool)
          n564 = Not Equal?(x=w1039, y=w1038) -> (x != y?=w1035:bool)
          n565 = Compound Arithmetic op=AND(w1037, w1036, w1035) -> (w1034:bool)
          n566 = case shown="True" w1034 {
            tunnel: w1041 -> [_ w1072]
            tunnel: w1040 -> [_ w1071]
            tunnel: [w1044 w1068] -> w1042
            tunnel: [w1044 w1067] -> w1043
            tunnel: w1039 -> [_ w1045]
            frame False {
              w1044 = ""
            }
            frame True {
              # "O2Eq"
              n567 = Fract/Exp String To Number(string=w1045) -> (number=w1046:dbl)  [unwired: 3 in, 1 out]
              n568 = Fract/Exp String To Number(string=w1072) -> (number=w1053:dbl)  [unwired: 3 in, 1 out]
              n569 = Fract/Exp String To Number(string=w1071) -> (number=w1049:dbl)  [unwired: 3 in, 1 out]
              n570 = Decrement(x=w1053) -> (x-1=w1054:dbl)
              n571 = Divide(x=w1046, y=20000.0) -> (x/y=w1047:dbl)
              n572 = Multiply(x=4.76, y=w1053) -> (x*y=w1058:dbl)
              n573 = Multiply(x=w1054, y=100.0) -> (x*y=w1056:dbl)
              n574 = Add(x=w1049, y=w1047) -> (x+y=w1050:dbl)
              n575 = Add(x=0.33, y=w1058) -> (x+y=w1060:dbl)
              n576 = Divide(x=w1056, y=w1060) -> (x/y=w1061:dbl)
              n577 = Subtract(x=w1050, y=w1061) -> (x-y=w1063:dbl)
              n578 = Multiply(x=w1063, y=2.0) -> (x*y=w1051:dbl)
              n579 = Divide(x=w1063, y=5.0) -> (x/y=w1052:dbl)
              n580 = Number To Fractional String(number=w1052, width (-)=i16 6, precision (6)=i16 3) -> (F-format string=w1067:string)  [unwired: 1 in]
              n581 = Number To Fractional String(number=w1051, width (-)=i16 6, precision (6)=i16 2) -> (F-format string=w1068:string)  [unwired: 1 in]
            }
          }
        }
        n582 = Replace Array Subset(array=w1032, new element #1=w1026, index (col) #1=5 ("disabled index (col)"), new element #2=w1025, index (col) #2=6 ("disabled index (col)")) -> (w1030:string[][])  [unwired: 2 in]
        n583 = local write "Sub-Cycle Pattern"(w1030) -> ()
      }
      frame "Total time calc" {
        w1087 = i16 2 ("width (-)")
        w1094 = ":"
        n584 = local read "Cycle Pattern"() -> (w1101:string[][])
        n585 = Index Array(array=w1101, index (col)=4 ("disabled index (col)")) -> (element=w1074:string[])  [unwired: 1 in]
        n586 = Array Size(array=w1074) -> (size(s)=w1076:i32)
        n587 = Search 1D Array(1D array=w1074, element="") -> (index of element=w1075:i32)  [unwired: 1 in]
        n588 = Equal?(x=w1075, y=-1) -> (x = y?=w1077:bool)
        n589 = Select(t=w1076, s=w1077, f=w1075) -> (s? t:f=w1073:i32)
        n590 = for {
          N: w1073 -> [_]
          tunnel: w1074 -> [w1109] mode=indexing
          shift-right: [w1111] -> w1097
          shift-left: 0 -> [w1112]
          n591 = xnode "Match Regular Expression"("input string"=w1109, "regular expression"=":" ("search string/char (-)")) -> ("before match"=w1108:string, "after match"=w1105:string)  [unwired: 4 in, 3 out]
          n592 = Decimal String To Number(string=w1108) -> (number=w1107:i32)  [unwired: 2 in, 1 out]
          n593 = Decimal String To Number(string=w1105) -> (number=w1104:i32)  [unwired: 2 in, 1 out]
          n594 = Multiply(x=w1107, y=60) -> (x*y=w1103:i32)
          n595 = Add(x=w1103, y=w1104) -> (x+y=w1102:i32)
          n596 = Add(x=w1102, y=w1112) -> (x+y=w1111:i32)
        }
        n597 = local read "Total Number of Cycles"() -> (w1098:T1)
        n598 = Multiply(x=w1097, y=w1098) -> (x*y=w1093:T1)
        n599 = Quotient & Remainder(x=w1093, y=3600.0) -> (x-y*floor(x/y)=w1080:T1, floor(x/y)=w1090:T1)
        n600 = Quotient & Remainder(x=w1080, y=60.0) -> (x-y*floor(x/y)=w1088:T1, floor(x/y)=w1089:T1)
        n601 = Number To Decimal String(number=w1090) -> (decimal integer string=w1095:string)  [unwired: 1 in]
        n602 = Number To Decimal String(number=w1089, width (-)=w1087) -> (decimal integer string=w1091:string)
        n603 = Number To Decimal String(number=w1088, width (-)=w1087) -> (decimal integer string=w1086:string)
        n604 = Concatenate Strings(w1095, w1094, w1091, w1094, w1086) -> (w1085:string)
        n605 = call <vilib>:"Search and Replace Pattern.vi"("string"=w1085, "regular expression (\"\")"=" " ("replace string (\"\")"), "replace string (\"\")"="0" ("replace string (\"\")"), "replace all? (F)"=TRUE) -> ("result string"=→"Total Test Duration (hrs)":string)  [unwired: 1 in, 1 out]
      }
      frame "update Cycle pattern " {
        n606 = local read "Cycle Pattern"() -> (w1240:string[][])
        n607 = Index Array(array=w1240, index (col)=1 ("disabled index (col)")) -> (element=w1225:string[])  [unwired: 1 in]
        n608 = String To Path(string=w1242) -> (path=w1243:path)
        n609 = Array Size(array=w1225) -> (size(s)=w1228:i32)
        n610 = Search 1D Array(1D array=w1225, element="") -> (index of element=w1227:i32)  [unwired: 1 in]
        n611 = List Folder(path=w1243, pattern="*.eyes") -> (filenames=w1241:string[])  [unwired: 2 in, 3 out]
        n612 = Equal?(x=w1227, y=-1) -> (x = y?=w1229:bool)
        n613 = Select(t=w1228, s=w1229, f=w1227) -> (s? t:f=w1226:i32)
        n614 = for {
          N: w1226 -> [_]
          tunnel: w1240 -> [w1259] mode=indexing
          tunnel: w1242 -> [w1252]
          tunnel: [w1254] -> w1235 mode=indexing
          tunnel: [w1256] -> w1239 mode=indexing
          tunnel: [w1253] -> w1236 mode=indexing
          tunnel: w1241 -> [w1251]
          tunnel: [w1246] -> w1232 mode=indexing
          n615 = Index Array(array=w1259, index #1=1 ("index"), index #2=3 ("index")) -> (element #1=w1250:string, element #2=w1255:string)
          n616 = Search 1D Array(1D array=w1251, element=w1250) -> (index of element=w1249:i32)  [unwired: 1 in]
          n617 = Not Equal?(x=w1249, y=-1) -> (x != y?=w1247:bool)
          n618 = case shown="True" w1247 {
            tunnel: [w1263 w1277] -> w1256
            tunnel: w1255 -> [_ w1273]
            tunnel: [w1263 w1271] -> w1254
            tunnel: [w1263 w1270] -> w1253
            tunnel: w1252 -> [_ w1269]
            tunnel: w1250 -> [w1262 w1268]
            tunnel: [w1261 w1268] -> w1246
            frame False {
              w1263 = "N/A" ("String")
              n619 = Concatenate Strings(w1262, " - File NOT AVAILABLE !!!" ("string")) -> (w1261:string)
            }
            frame True {
              w1281 = i16 2 ("width (-)")
              n620 = Concatenate Strings(w1269, w1268) -> (w1299:string)
              n621 = String To Path(string=w1299) -> (path=w1298:path)
              n622 = call <vilib>:"Search and Replace Pattern.vi"("string"=w1273, "regular expression (\"\")"="[a-x ]" ("format string"), "replace string (\"\")"="", "replace all? (F)"=TRUE) -> ("result string"=w1270:string)  [unwired: 1 in, 1 out]
              n623 = call-poly <vilib>:"Read From Spreadsheet File.vi"("file path (dialog if empty)"=w1298) -> ("first row"=w1267:string[])  [unwired: 6 in, 4 out]
              n624 = Delete From Array(array=w1267, length=1, index=0) -> (array with subset deleted=w1266:string[])  [unwired: 1 out]
              n625 = Array Size(array=w1266) -> (size(s)=w1297:i32)
              n626 = Equal?(x=w1270, y="") -> (x = y?=w1285:bool)
              n627 = Subtract(x=w1297, y=12) -> (x-y=w1295:i32)
              n628 = Select(t="0", s=w1285, f=w1270) -> (s? t:f=w1284:string)
              n629 = Index Array(array=w1266, index=w1295) -> (element=w1271:string)
              n630 = Decimal String To Number(string=w1284) -> (number=w1294:i32)  [unwired: 2 in, 1 out]
              n631 = Decimal String To Number(string=w1271) -> (number=w1293:i32)  [unwired: 2 in, 1 out]
              n632 = Multiply(x=w1294, y=w1293) -> (x*y=w1292:i32)
              n633 = Quotient & Remainder(x=w1292, y=60) -> (x-y*floor(x/y)=w1290:i32, floor(x/y)=w1289:i32)
              n634 = Number To Decimal String(number=w1290, width (-)=w1281) -> (decimal integer string=w1287:string)
              n635 = Number To Decimal String(number=w1289, width (-)=w1281) -> (decimal integer string=w1286:string)
              n636 = Concatenate Strings(w1286, ":", w1287) -> (w1280:string)
              n637 = call <vilib>:"Search and Replace Pattern.vi"("string"=w1280, "regular expression (\"\")"=" " ("replace string (\"\")"), "replace string (\"\")"="0" ("replace string (\"\")"), "replace all? (F)"=TRUE) -> ("result string"=w1277:string)  [unwired: 1 in, 1 out]
            }
          }
        }
        n638 = Replace Array Subset(array=w1240, new element #1=w1232, index (col) #1=1 ("disabled index (col)"), new element #2=w1235, index (col) #2=2 ("disabled index (col)"), new element #3=w1236, index (col) #3=3 ("disabled index (col)"), new element #4=w1239, index (col) #4=4 ("disabled index (col)")) -> (w1244:string[][])  [unwired: 4 in]
        n639 = local write "Cycle Pattern"(w1244) -> ()
      }
      frame "load cycle name" {
        n640 = property on="Cycle Pattern" class="Tbl (strict)"() -> ("EditPos"=w1305:T3)  [unwired: 2 in, 2 out]
        n641 = Unbundle By Name(w1305) -> ("Row"=w1303:i32, "Column"=w1302:i32)
        n642 = local read "Cycle Pattern"() -> (w1301:string[][])
        n643 = call "SubCycles list.vi"() -> ("Subcycle name"=w1304:string)  [unwired: 10 in, 1 out]
        n644 = Replace Array Subset(array=w1301, new element=w1304, index (row)=w1303, index (col)=w1302) -> (w1300:string[][])
        n645 = local write "Cycle Pattern"(w1300) -> ()
      }
      frame "load test array" {
        n646 = local read "Total Test Duration (hrs)"() -> (w1313:T8)
        n647 = local read "Cycle Name"() -> (w1309:T5)
        n648 = Equal?(x=w1309, y="") -> (x = y?=w1308:bool)
        n649 = Not Equal?(x=w1313, y="0:00:00") -> (x != y?=w1307:bool)
        n650 = Or(x=w1307, y=w1308) -> (x .or. y?=w1306:bool)
        n651 = case shown="True" w1306 {
          selector: w1306 -> [w1314 _]
          tunnel: [FALSE TRUE] -> w1311
          frame False {
            n652 = case shown="False" w1314 {
              frame False {
                n653 = One Button Dialog(message="Incomplete Data!\nReview the cycle pattern!") -> ()  [unwired: 1 in, 1 out]
              }
              frame True {
              }
            }
          }
          frame True {
            w1320 = 0.0 ("default (0 I32)")
            n654 = local read "Cycle Name"() -> (w1335:T5)
            n655 = Concatenate Strings("C:\\Setup Files\\Cycles Folder\\", w1335, ".eyec" ("string")) -> (w1333:string)
            n656 = String To Path(string=w1333) -> (path=w1334:path)
            n657 = local read "Total Number of Cycles"() -> (w1331:T1)
            n658 = call-poly <vilib>:"Read From Spreadsheet File.vi"("file path (dialog if empty)"=w1334) -> ("first row"=w1317:string[])  [unwired: 6 in, 4 out]
            n659 = call "Remove names.vi"("Array in"=w1317) -> ("Array out"=w1326:string[])  [unwired: 10 in]
            n660 = Index Array(array=w1317, index #1=14 ("index"), index #2=15 ("index")) -> (element #1=w1322:string, element #2=w1318:string)
            n661 = Number To Decimal String(number="Ageing Gas") -> (decimal integer string=w1330:string)  [unwired: 1 in]
            n662 = Number To Decimal String(number=w1331) -> (decimal integer string=w1329:string)  [unwired: 1 in]
            n663 = Decimal String To Number(string=w1318, default (0L)=w1320) -> (number=w1319:dbl)  [unwired: 1 in, 1 out]
            n664 = Decimal String To Number(string=w1322, default (0L)=w1320) -> (number=w1321:dbl)  [unwired: 1 in, 1 out]
            n665 = property on="Inlet temp Age" class="DigNum (strict)"("Value"=w1321) -> ()  [unwired: 2 in, 2 out]
            n666 = property on="Flow rate Age" class="DigNum (strict)"("Value"=w1319) -> ()  [unwired: 2 in, 2 out]
            n667 = Build Array (concatenate)(w1330, w1329, w1326) -> (w1325:string[])
            n668 = shared-variable "cRIO-9082\\Library 1.lvlib\\Ageing Variables"(w1325) -> ()  [unwired: 1 in, 1 out]
          }
        }
        "Test Compiled" <- w1311
      }
      frame "convert to num" {
        n669 = local read "EditPos Subc"() -> (w1340:T3)
        n670 = Unbundle By Name(w1340) -> ("Row"=w1341:i32, "Column"=w1338:i32)
        n671 = Equal?(x=w1338, y=7) -> (x = y?=w1337:bool)
        n672 = case shown="False" w1337 {
          tunnel: w1341 -> [_ w1346]
          tunnel: w1338 -> [_ w1344]
          tunnel: w1340 -> [_ _]
          frame True {
          }
          frame False {
            n673 = local read "Sub-Cycle Pattern"() -> (w1343:string[][])
            n674 = call "Conv to num.vi"("Column"=w1344, "Row"=w1346, "Array"=w1343) -> ("result string"=w1345:string)  [unwired: 8 in]
            n675 = Replace Array Subset(array=w1343, new element=w1345, index (row)=w1346, index (col)=w1344) -> (w1342:string[][])
            n676 = local write "Sub-Cycle Pattern"(w1342) -> ()
          }
        }
      }
      frame "check scycle name" {
        n677 = local read "Sub-Cycle Name"() -> (w1347:T5)
        n678 = call <vilib>:"Search and Replace Pattern.vi"("string"=w1347, "regular expression (\"\")"="[^0-9a-zA-Z ]" ("format string"), "replace string (\"\")"="", "replace all? (F)"=TRUE) -> ("result string"=w1353:string)  [unwired: 1 in, 1 out]
        n679 = Not Equal?(x=w1353, y=w1347) -> (x != y?=w1352:bool)
        n680 = case shown="False" w1352 {
          tunnel: w1353 -> [w1354 w1355]
          tunnel: [w1354 w1355] -> w1348
          frame False {
          }
          frame True {
            n681 = One Button Dialog(message="Unsuitable character for the file name!") -> ()  [unwired: 1 in, 1 out]
          }
        }
        n682 = local write "Sub-Cycle Name"(w1348) -> ()
      }
      frame "check cycle name" {
        n683 = local read "Cycle Name"() -> (w1357:T5)
        n684 = call <vilib>:"Search and Replace Pattern.vi"("string"=w1357, "regular expression (\"\")"="[^0-9a-zA-Z ]" ("format string"), "replace string (\"\")"="", "replace all? (F)"=TRUE) -> ("result string"=w1363:string)  [unwired: 1 in, 1 out]
        n685 = Not Equal?(x=w1363, y=w1357) -> (x != y?=w1362:bool)
        n686 = case shown="False" w1362 {
          tunnel: w1363 -> [w1364 w1365]
          tunnel: [w1364 w1365] -> w1358
          frame False {
          }
          frame True {
            n687 = One Button Dialog(message="Unsuitable character for the file name!") -> ()  [unwired: 1 in, 1 out]
          }
        }
        n688 = local write "Cycle Name"(w1358) -> ()
      }
      frame "Multigas connect" {
        # "add here logic to verify the user requirements and the machine state\n0 - not connected\n1 - MKS1 & Ext An Up\n2 - MKS2 & Ext An Dn\n3 - MKS 1 & 2  & Ext An Up & Dn"
        n689 = flat-sequence {
          frame #0 {
            "Connected?" <- TRUE
          }
        }
      }
      frame "Multigas disconnect" {
      }
    }
    n690 = local read "stop 2"() -> (w743:bool)
  }
  n691 = node-c288(w1) -> ()  [unwired: 1 out]
  n692 = local write "stop 2"(w11) -> ()
  n693 = disable-structure shown="Disabled" {
    frame Disabled {
      n694 = while {
        tunnel: [w1406] -> w1391
        tunnel: [w1405] -> w1390
        stop <- w1402 stop-if-true
        n695 = TCP Open Connection(address="192.168.1.3", remote port or service name=u16 7700) -> (connection ID=w1406:refnum<k5>, error out=w1405:errorcluster)  [unwired: 3 in]
        n696 = Unbundle By Name(w1405) -> ("status"=w1407:bool)
        n697 = Not(x=w1407) -> (.not. x?=w1403:bool)
        n698 = Or(x=w1403, y="stop TCP") -> (x .or. y?=w1402:bool)
      }
      n699 = Concatenate Strings("\r", "\n") -> (w1379:string)
      n700 = Concatenate Strings("MSSM,0,1,1" ("data in"), w1379) -> (w1386:string)
      n701 = TCP Write(connection ID=w1391, data in=w1386, error in (no error)=w1390) -> (connection ID out=w1394:refnum<k5>, error out=w1395:errorcluster)  [unwired: 1 in, 1 out]
      n702 = Concatenate Strings("MSMD,1,7,1,1,1,1,2,1,1,3,1,1,4,1,1,5,1,1,6,1,1,7,1" ("data in"), w1379) -> (w1381:string)
      n703 = TCP Write(connection ID=w1394, data in=w1381, error in (no error)=w1395) -> (connection ID out=w1392:refnum<k5>, error out=w1393:errorcluster)  [unwired: 1 in, 1 out]
      n704 = Concatenate Strings("MSTT,1,0" ("string"), w1379) -> (w1380:string)
      n705 = TCP Write(connection ID=w1392, data in=w1380, error in (no error)=w1393) -> (connection ID out=w1378:refnum<k5>, error out=w1377:errorcluster)  [unwired: 1 in, 1 out]
      n706 = UDP Open(9:500 ("timeout ms (25000)"), 11:u16 7701 ("port")) -> ()  [unwired: 3 in, 3 out]
      n707 = UDP Read(timeout ms (25000)=500) -> (data out=w1369:string)  [unwired: 3 in, 4 out]
      n708 = while {
        shift-right: [w1398] -> _
        shift-left: w1369 -> [w1401]
        tunnel: [w1399] -> w1370 mode=indexing
        stop <- w1396 stop-if-true
        n709 = Search/Split String(string=w1401, search string/char (-)=",") -> (substring before match=w1399:string, match + rest of string=w1398:string)  [unwired: 1 in, 1 out]
        n710 = String Length(string=w1398) -> (length=w1397:i32)
        n711 = Equal To 0?(x=w1397) -> (x = 0?=w1396:bool)
      }
      n712 = call "7170string to array.vi"("Array in"=w1370) -> ()  [unwired: 4 in, 1 out]
      n713 = UDP Close() -> ()  [unwired: 2 in, 2 out]
      n714 = Concatenate Strings("MSTP,0,0" ("string"), "\r", "\n") -> (w1373:string)
      n715 = TCP Write(data in=w1373) -> (connection ID out=w1375:refnum<k5>, error out=w1376:errorcluster)  [unwired: 3 in, 1 out]
      n716 = TCP Close Connection(connection ID=w1375, error in (no error)=w1376) -> ()  [unwired: 1 in, 2 out]
    }
    frame Enabled {
    }
  }
  n717 = node-c288(w8) -> ()  [unwired: 1 out]
  "Table" <- string[][] [] ("Table")
